vi "eyecat MAX v2-1_JS_160202.vi"() -> ()   [LabVIEW 2014]
doc: "This VI is an upgrade from the WIN 1_v4 that implements the ageing subrutine"
uses:
  Buttons/String output.ctl
  <vilib>/Utility/miscctls.llb/LVRowAndColumnTypeDef.ctl
  Buttons/Numeric control.ctl
  Buttons/String input.ctl
  Buttons/Numeric indicator.ctl
  Controls Win/Control 3.ctl
  <vilib>/Platform/TimedLoop/XDataNode/nitl_modes.ctl
  <vilib>/Platform/TimedLoop/XDataNode/timing_clust.ctl
  <vilib>/Platform/TimedLoop/XDataNode/wakeup.ctl
  <vilib>/Utility/file.llb/Write To Spreadsheet File (string).vi
  <vilib>/Utility/file.llb/Read From Spreadsheet File (string).vi
  <vilib>/Utility/file.llb/Read From Spreadsheet File (DBL).vi
  <vilib>/regexp/Match Regular Expression.xnode
  <vilib>/Platform/TimedLoop/XDataNode/XDataNode.xnode
  <vilib>/Platform/TimedLoop/XDataNode/XDNodeRunTimeDep.lvlib
panel:
  in  "Alarm":bool
  in  "Analyser":bool
  in  "MFC":bool
  in  "System":bool
  in  "Ageing":bool
  in  "Performance":bool
  in  "Home":bool
  out "NO":dbl[](array[numeric])
  out "CO":dbl[](array[numeric])
  out "MKS":bool
  out "7170":bool
  out "Pressure":dbl
  in  "Duration -1":i32
  in  "Demo Sync":i32
  in  "Demo On":bool
  in  "FlowGuide":bool
  in  "Mean(Off)/Interval(On) 2":bool
  in  "Flow Band %":dbl=1.04
  in  "Flow Sync":i32
  in  "Execute Leak Test Button":bool
  out "Emissions":dbl[](array[numeric])
  in  "Temperature Sync":i32
  in  "TempGuide":bool
  in  "Temp Band %":dbl=1.04
  in  "Mean(Off)/Interval(On)":bool
  in  "MKS 5Hz":bool
  out "output cluster":T2
  out "Lambda":dbl[](array[numeric])
  out "MKS HC":dbl
  in  "HC Index":i32
  in  "MFC Number":i32
  out "Open/Closed \nLoop":dbl[](array[numeric])
  out "Air Cyc 2":dbl[](array[numeric])
  in  "Cycle size":i32
  out "MFC Setpoint/Delivery":dynamicdata(graph)
  out "ExtAnDn":bool
  out "ExtAnUp":bool
  out "HC Cyc 2":dbl[](array[numeric])
  out "SO Valve 2":dbl[](array[numeric])
  out "SO Valve 1":dbl[](array[numeric])
  out "Air Bal":dbl[](array[numeric])
  out "HC Bal":dbl[](array[numeric])
  out "Air Cyc 1":dbl[](array[numeric])
  out "HC Cyc 1":dbl[](array[numeric])
  out "File name":string
  out "Log?":bool
  out "Advanced Logging":bool
  out "Connected":bool
  out "Furnace temp 2":dbl
  out "Full system?":bool
  out "Log interval (seconds)":T1
  in  "Flow rate Age":dbl
  in  "Inlet temp Age":dbl
  out "Stopped?":bool
  in  "Stop Cmd":T1
  out "Connected?":bool
  out "Error":dbl
  out "Iteration Duration":i64
  out "Finished Late? [i-1]":bool
  out "Furnace temp 1":dbl
  out "stop 2":bool
  in  "Enum 1":i16=1
  in  "Acknowledge":bool
  out "Test number":u16
  out "Flag1":bool=TRUE
  out "EditPos Subc":T3
  out "Flag 2":bool=TRUE
  in  "Tab Control":T4(tab)
  out "Warm Up":bool
  in  "Leak Test":bool
  in  "Stop Test":bool
  in  "Log Test Data":bool
  in  "Start Test":bool
  in  "Adv Settings":bool
  out "Doors Unlocked":bool
  in  "Temperature Limit (°C)":T1=1200.0 min=0.0 max=1200.0 step=1.0
  in  "File Name":T5="Test"
  in  "File Path":path=path "C:/DATA LOG"
  out "Fail":bool
  out "Pass":bool
  in  "Select Test Type":T6(radio)
  out "Standby":bool
  out "Doors Open":bool
  out "Extractor Fan On":bool
  out "Test In Progress":bool
  out "Cool Down":bool
  out "System Alarm":bool
  in  "Inlet Temperature (°C)":T1=400.0 min=350.0 max=1000.0 step=1.0
  in  "Inlet LAMBDA Rich":T1=0.9 min=0.85 max=0.96 step=0.001
  in  "Inlet LAMBDA Lean":T1=1.2 min=1.02 max=3.0 step=0.001
  in  "Test Stop temperature (°C)":T1=300.0 min=100.0 max=1000.0 step=1.0
  in  "Test Start Temperature (°C)":T1=125.0 min=0.0 max=500.0 step=1.0
  in  "Furnace Ramp Rate (°C/min)":T1=15.0 min=1.0 max=50.0 step=0.1
  in  "NO:CO Ratio":T1=1.1 min=1.0 max=5.0 step=0.1
  in  "Inlet O2 (%)":T1=0.5 min=0.0 max=14.0 step=0.01
  in  "Inlet LAMBDA":T1=1.0 min=0.6 max=3.0 step=0.001
  out "Space Velocity (h-1)":T7
  out "Vol Flow @ STP (l/min)":T7
  in  "Test Flow Rate(g/s)":T1 min=0.0 max=100.0 step=0.01
  out "Sample Volume (litres)":T7
  in  "Number of Samples":T1=1.0 min=1.0 max=6.0 step=1.0
  in  "Sample Diameter (mm)":T1
  out "CO Theory (%)":T7 format="%#_3g"
  out "CO Theory (%)":T7 format="%#_3g"
  out "HC Theory (%)":T7
  in  "Sample Length (mm)":T1 min=0.0 step=0.5
  in  "NO ppm SW":dbl=500.0 caption="NO (ppm)" min=0.0 max=500.0 step=1.0
  in  "NO ppm Loff":T1 caption="NO ppm"
  in  "Delete sCycle":bool
  in  "Load sCycle":bool
  in  "Save sCycle":bool
  in  "Clear subcycle":bool
  in  "Clear Cycle Pattern":bool
  in  "Save Cycle":bool
  in  "Load Cycle":bool
  in  "Delete Cycle":bool
  out "Test Compiled":bool
  in  "Compile Test Button":bool
  in  "Sub-Cycle List":i32(listbox)=1
  in  "Cycle List":i32(listbox)=2
  out "Total Test Duration (hrs)":T8
  in  "Ageing Gas":enum32{"Radio Selection 1", "Radio Selection 2"}(radio)
  in  "Sub-Cycle Pattern":string[][](table) caption="Subcycle pattern"
  in  "Total Number of Cycles":T1=1.0 min=1.0 max=10000.0 step=1.0
  in  "Cycle Pattern":string[][](table)
  in  "Sub-Cycle Name":T5
  in  "Cycle Name":T5
  out "Heat Exchanger Temperatures (°C)":dynamicdata(graph)
  out "Flow Rate (g/s)":dynamicdata(graph)
  out "Sample Temperatures (°C)":dynamicdata(graph)
  out "System Temperatures (°C)":dynamicdata(graph)
  in  "Graph 1 Box":string(combo)="CO"
  in  "Graph 4 Box":string(combo)="NO"
  in  "Graph 3 Box":string(combo)="Air Cycle 1"
  in  "Graph 2 Box":string(combo)="HC Cycle 1"
  out "MFC Graph 4":dynamicdata(graph)
  out "MFC Graph 3":dynamicdata(graph)
  out "MFC Graph 1":dynamicdata(graph)
  out "MFC Graph 2":dynamicdata(graph)
  out "HC Concentration (ppm)":dynamicdata(graph)
  out "Lambda":dynamicdata(graph)
  out "O2/CO Concentration":dynamicdata(graph)
  out "NO Concentration (ppm)":dynamicdata(graph)
  in  "Purge System":bool
  in  "Alarm ack":bool
  in  "Clear log":bool
  out "Table":string[][](table)
  out "Soft Alarm":bool
  out "Hard Alarm":bool
  # "0 CO \n1 HC Cyc 1\n2 Air Cyc 1\n3 NO\n4 Air Bal\n5 HC Bal\n6 Air Cyc 2\n7 HC Cyc 2"
  # "1% = 0.01"
  # "Test Type"
  # "Test Commands"
  # "System Indicators"
  # "Leak Test"
  # "Catalyst Specification"
  # "Lightoff Settings"
  # "Furnace Lightoff Settings"
  # "Sweep Settings"
  # "CO/HC Lightoff Settings"
  # "0.96 < lambda < 0.85"
  # "1.02< lambda < 1.6"
  # "350 < Tinlet < 1000"
  # "NO Lightoff Settings"
  # "Flow Specification"
  # "Cycle Compiled"
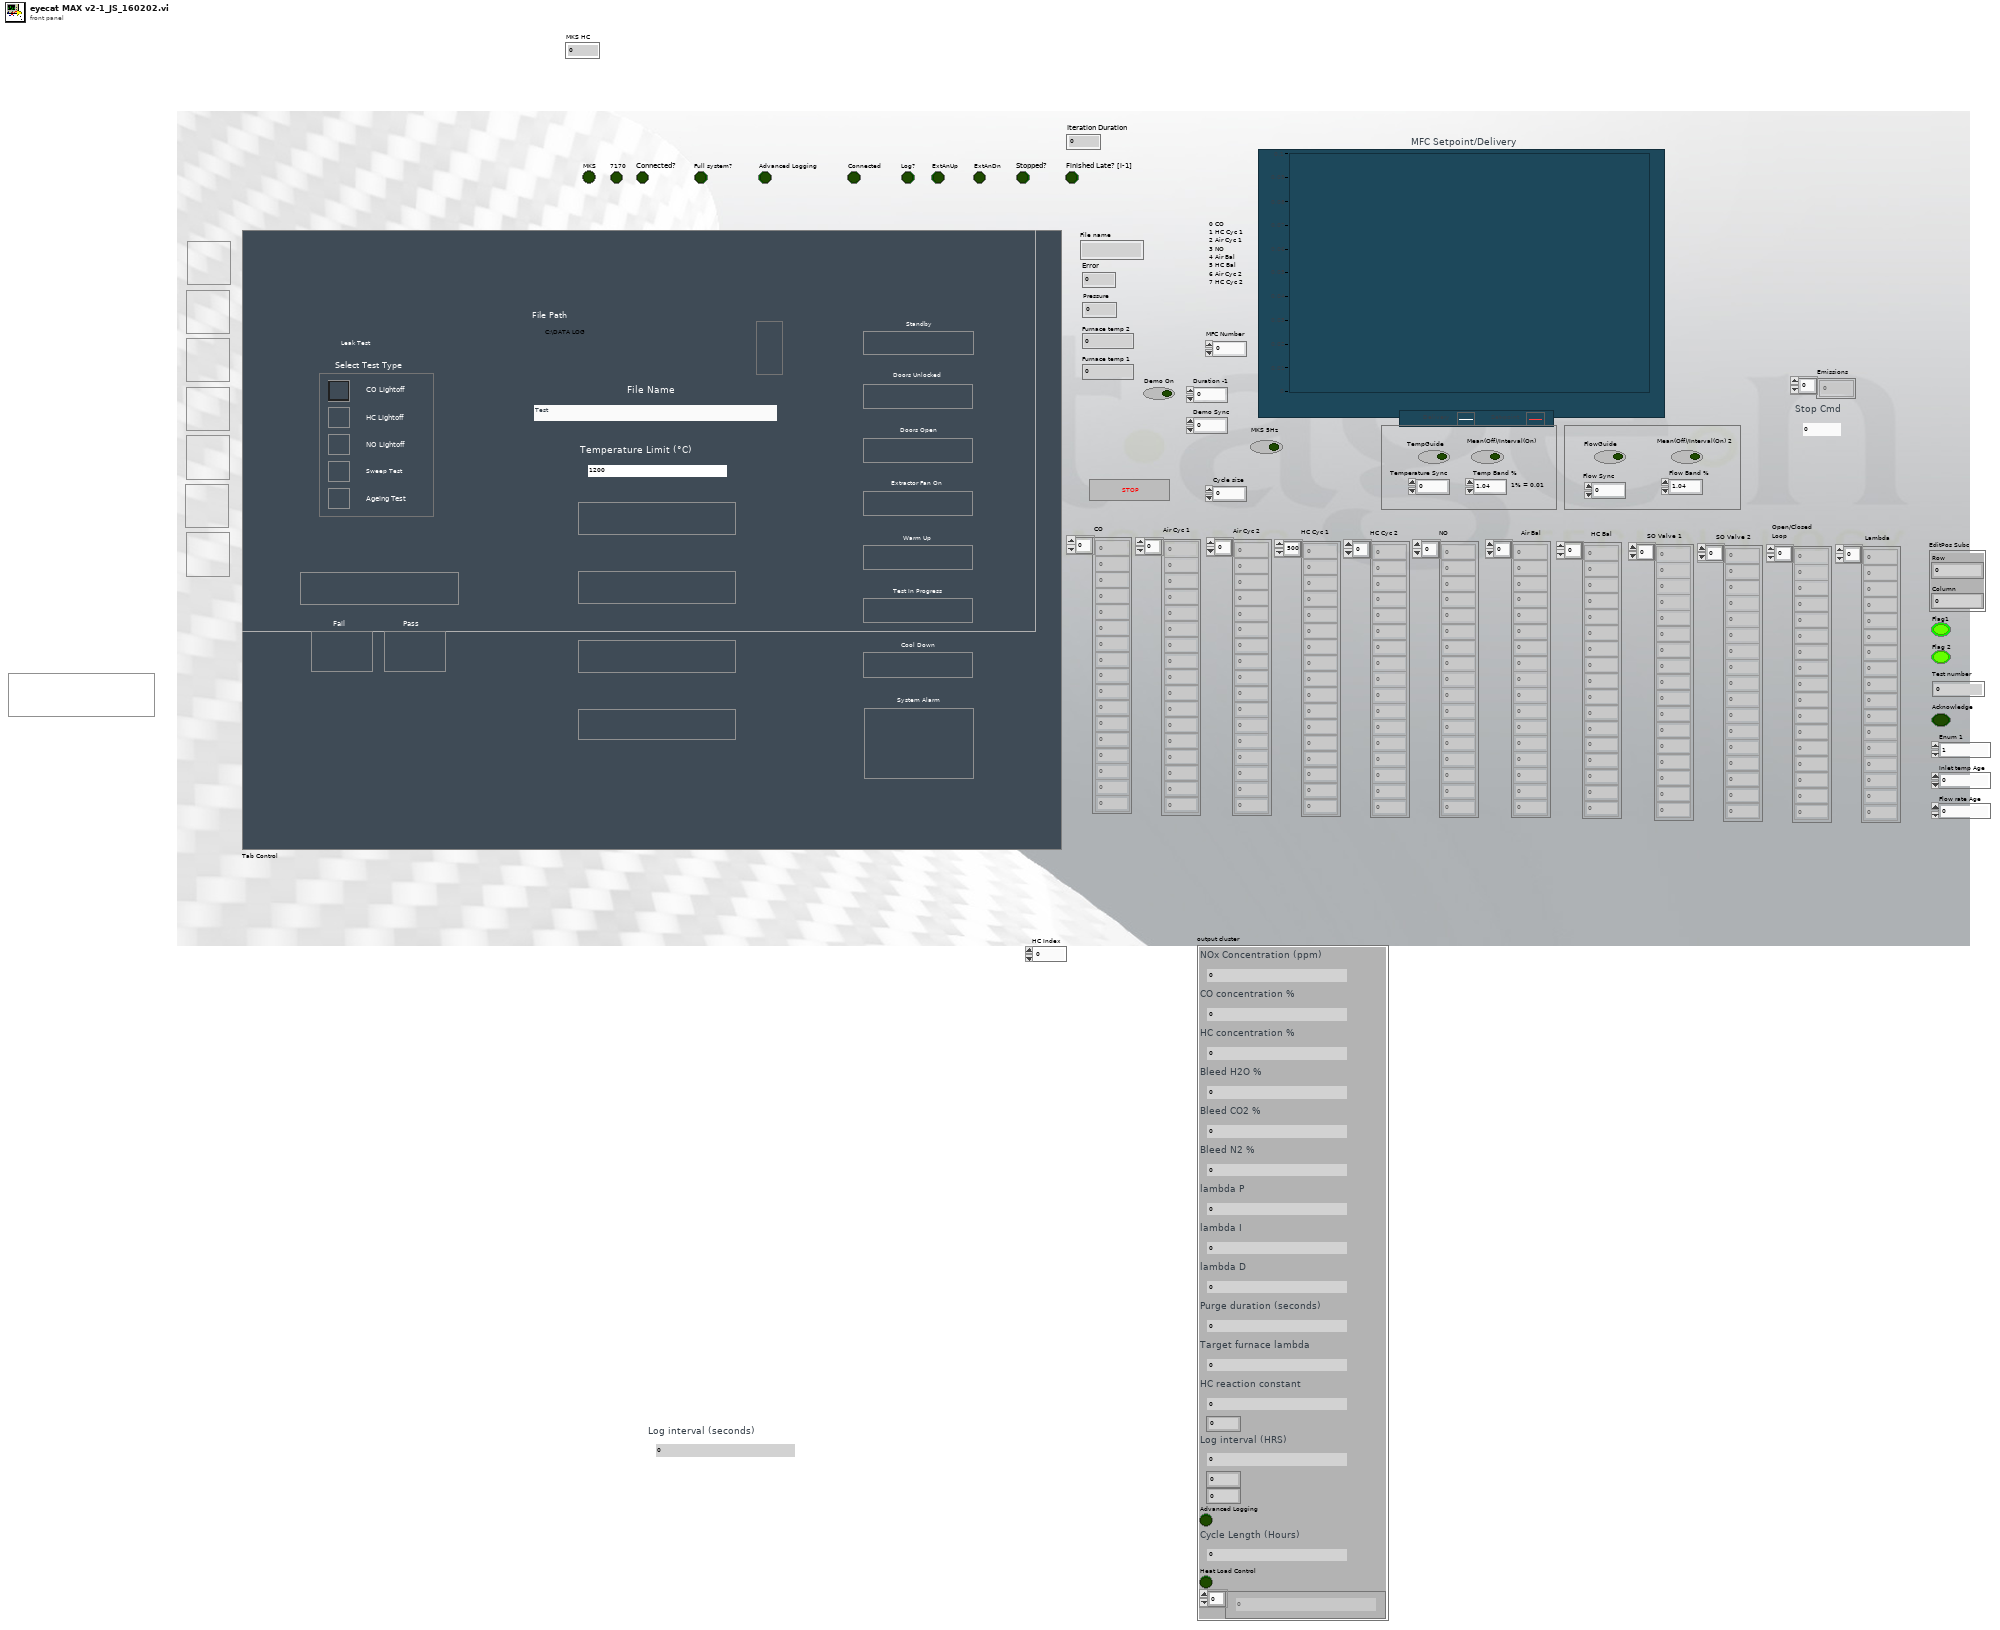
[diagram p1: front panel]
types:
  T1 = typedef "Numeric control.ctl" = dbl
  T2 = cluster{"NOx Concentration (ppm)":T1, "CO concentration %":T1, "HC concentration %":T1, "Bleed H2O %":T1, "Bleed CO2 %":T1, "Bleed N2 %":T1, "lambda P":T1, "lambda I":T1, "lambda D":T1, "Purge duration (seconds)":T1, "Target furnace lambda":T1, "HC reaction constant":T1, i16, "Log interval (HRS)":T1, i16, i16, "Advanced Logging":bool, "Cycle Length (Hours)":T1, "Heat Load Control":bool, T1[]}
  T3 = typedef "LVRowAndColumnTypeDef.ctl" = cluster{"Row":i32, "Column":i32}
  T4 = enum32{"MAIN", "PERFORMANCE TEST SETUP", "AGEING TEST SETUP", "SYSTEM DATA", "MFC", "ANALYSER DATA", "ALARM LOG"}
  T5 = typedef "String input.ctl" = string
  T6 = enum32{"CO Lightoff", "HC Lightoff", "NO Lightoff", "Sweep Test", "Ageing Test"}
  T7 = typedef "Numeric indicator.ctl" = dbl
  T8 = typedef "String output.ctl" = string
  T9 = typedef "XDNodeRunTimeDep.lvlib/nitl_modes.ctl" = enum32{"No Change", "Process missed periods, maintain original phase", "Discard missed periods, maintain original phase", "Process missed periods, ignore original phase", "Discard missed periods, ignore original phase"}
  T10 = typedef "Control 3.ctl" = enum16{"main", "start test", "save subc", "load subc", "delete subc", "clear table 1", "update list 1", "save cycle", "load cycle", "delete cycle", "clear table 2", "update list 2", "calc HC CO", "Total time calc", "update Cycle pattern ", "load cycle name", "convert to num", "load test array", "check scycle name", "check cycle name", "Multigas connect", "Multigas disconnect", "Leak Test"}
  T11 = enum8{"Enabled", "Disabled", "Disabled and Grayed Out"}
  T12 = typedef "XDNodeRunTimeDep.lvlib/timing_clust.ctl" = cluster{"Expected End [f-1]":u64, "Actual End [f-1]":u64, "Finished Late? [f-1]":bool, "Expected End [i-1]":u64, "Actual End [i-1]":u64, "Finished Late? [i-1]":bool, "Expected Start [i]":u64, "Actual Start [i]":u64, "Expected Start [f]":u64, "Actual Start [f]":u64, "Source Name":string, "Structure Name":string, "Period":i64, "Deadline":i64, "Offset":i64, "Start":i64, "Priority":i32, "Timeout":i32, "Mode":T9, "Wakeup Reason":T13, "Error":errorcluster, "Source Type":string, "Secondary Source Type":string, "Global End Time":u64, "Global Start Time":u64, "Frame Duration":u64, "Iteration Duration":u64, "Assigned CPU":i32, "I/O Scan Engine Mode":u32}
  T13 = typedef "XDNodeRunTimeDep.lvlib/wakeup.ctl" = enum32{"Normal", "Aborted", "Asynchronous wakeup", "Timing source error", "Timed loop error", "Timeout"}
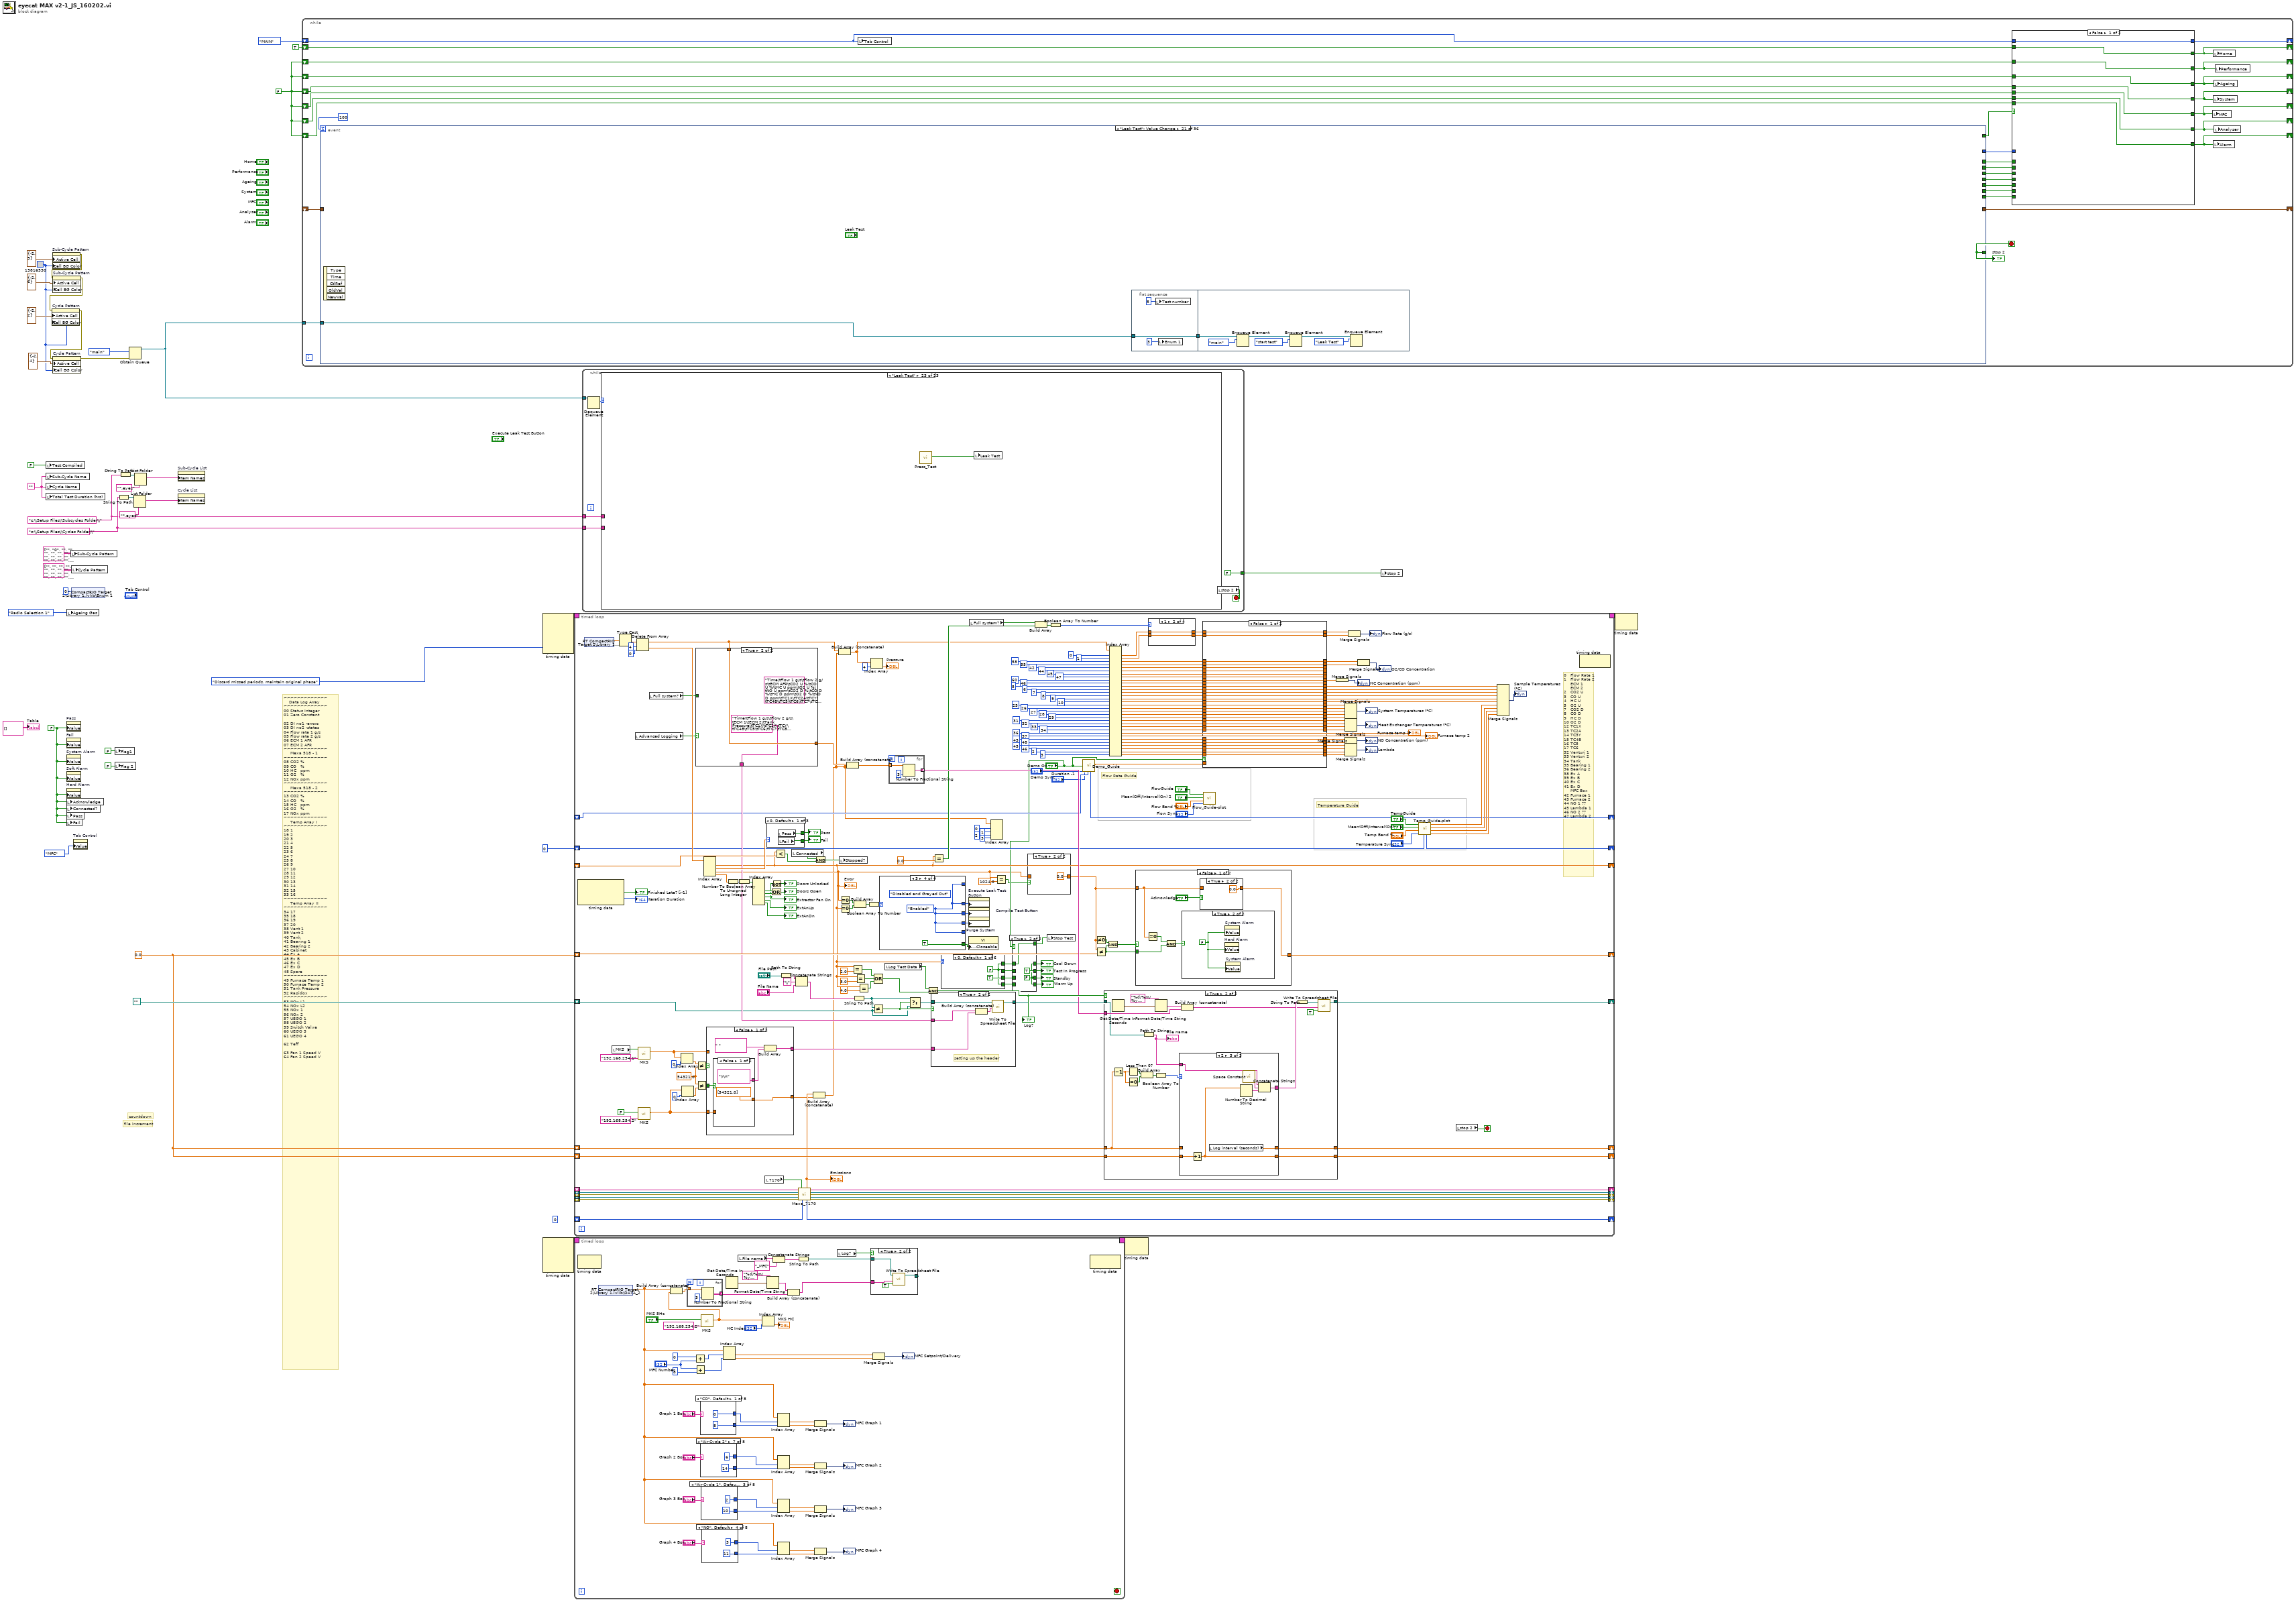
[diagram p0: block diagram]
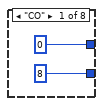
[diagram p2: hidden frame]
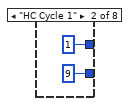
[diagram p3: hidden frame]
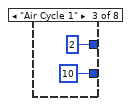
[diagram p4: hidden frame]
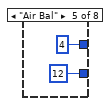
[diagram p5: hidden frame]
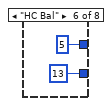
[diagram p6: hidden frame]
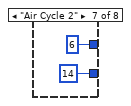
[diagram p7: hidden frame]
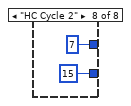
[diagram p8: hidden frame]
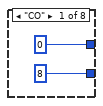
[diagram p9: hidden frame]
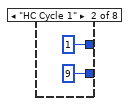
[diagram p10: hidden frame]
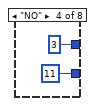
[diagram p11: hidden frame]
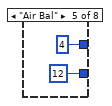
[diagram p12: hidden frame]
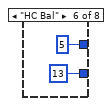
[diagram p13: hidden frame]
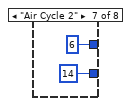
[diagram p14: hidden frame]
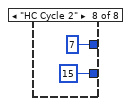
[diagram p15: hidden frame]
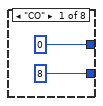
[diagram p16: hidden frame]
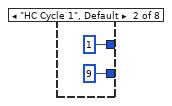
[diagram p17: hidden frame]
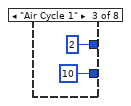
[diagram p18: hidden frame]
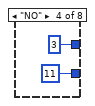
[diagram p19: hidden frame]
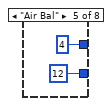
[diagram p20: hidden frame]
diagram:
  w1 = FALSE
  (unwired) 0 ("index")
  w9 = FALSE
  w8 = 0.0 ("y")
  w24 = ""
  w27 = "c:\\Setup Files\\Cycles Folder\\"
  w33 = u32 13816530
  w25 = "c:\\Setup Files\\Subcycles Folder\\"
  # "~~~~~~~~~~~~~\n    Data Log Array\n~~~~~~~~~~~~~\n00 Status Integer\n01 Zero Constant\n\n02 DI no1 -errors\n03 DI no2 -states\n04 Flow rate 1 g/s\n05 Flow rate 2 g/s\n06 ECM 1 AFR\n07 ECM 2 AFR\n~~~~~~~~~~~~~\n     Mexa 518 - 1\n~~~~~~~~~~~~~\n08 CO2 %\n09 CO   %\n10 HC   ppm\n11 O2   %\n12 NOx ppm\n~~~~~~~~~~~~~\n     Mexa 518 - 2\n~~~~~~~~~~~~~\n13 CO2 %\n14 CO   %\n15 HC   ppm\n16 O2   %\n17 NOx ppm\n~~~~~~~~~~~~~\n     Temp Array I\n~~~~~~~~~~~~~\n18 1\n19 2 \n20 3\n21 4\n22 5\n23 6\n24 7\n25 8\n26 9\n27 10\n28 11\n29 12\n30 13\n31 14\n32 15\n33 16\n~~~~~~~~~~~~~\n     Temp Array II\n~~~~~~~~~~~~~\n34 17\n35 18\n36 19\n37 20\n38 Vent 1\n39 Vent 2\n40 Tank\n41 Bearing 1\n42 Bearing 2\n43 Cabinet\n44 Ex A\n45 Ex B\n46 Ex C\n47 Ex D\n48 Spare\n~~~~~~~~~~~~~\n49 Furnace Temp 1\n50 Furnace Temp 2\n51 Tank Pressure\n52 Rapidox\n~~~~~~~~~~~~~\n53 NOx L1\n54 NOx L2\n55 NOx 1\n56 NOx 2\n57 UEGO 1\n58 UEGO 2\n59 Switch Valve\n60 UEGO 3\n61 UEGO 4\n\n62 Teff\n\n63 Fan 1 Speed V\n64 Fan 2 Speed V"
  # "file increment"
  # "countdown"
  n1 = local write "Test Compiled"(FALSE ("Cycle Compiled")) -> ()
  n2 = local write "Sub-Cycle Name"(w24) -> ()
  n3 = local write "Cycle Name"(w24) -> ()
  n4 = local write "Total Test Duration (hrs)"(w24) -> ()
  n5 = property on="Sub-Cycle Pattern" class="Tbl (strict)"("Active Cell"=T3 {"Row"=-2, "Column"=5} ("Active Cell:Active Cell"), "Cell BG Color"=w33) -> (error out=w38:errorcluster)  [unwired: 2 in, 1 out]
  n6 = property on="Sub-Cycle Pattern" class="Tbl (strict)"(error in=w38, "Active Cell"=T3 {"Row"=-2, "Column"=6} ("Active Cell:Active Cell"), "Cell BG Color"=w33) -> (error out=w37:errorcluster)  [unwired: 1 in, 1 out]
  n7 = property on="Cycle Pattern" class="Tbl (strict)"(error in=w37, "Active Cell"=T3 {"Row"=-2, "Column"=2} ("Active Cell:Active Cell"), "Cell BG Color"=w33) -> (error out=w35:errorcluster)  [unwired: 1 in, 1 out]
  n8 = property on="Cycle Pattern" class="Tbl (strict)"(error in=w35, "Active Cell"=T3 {"Row"=-2, "Column"=4} ("Active Cell:Active Cell"), "Cell BG Color"=w33) -> (error out=w32:errorcluster)  [unwired: 1 in, 1 out]
  n9 = property on="Pass" class="Bool (strict)"("Value"=w9) -> ()  [unwired: 2 in, 2 out]
  n10 = property on="Fail" class="Bool (strict)"("Value"=w9) -> ()  [unwired: 2 in, 2 out]
  n11 = property on="System Alarm" class="Bool (strict)"("Value"=w9) -> ()  [unwired: 2 in, 2 out]
  n12 = property on="Soft Alarm" class="Bool (strict)"("Value"=w9) -> ()  [unwired: 2 in, 2 out]
  n13 = property on="Hard Alarm" class="Bool (strict)"("Value"=w9) -> ()  [unwired: 2 in, 2 out]
  n14 = local write "Acknowledge"(w9) -> ()
  n15 = local write "Connected?"(w9) -> ()
  n16 = local write "Pass"(w9) -> ()
  n17 = local write "Fail"(w9) -> ()
  n18 = local write "Ageing Gas"(enum32{"Radio Selection 1", "Radio Selection 2"}."Radio Selection 1" ("Ageing Gas")) -> ()
  n19 = local write "Sub-Cycle Pattern"(string[][] [["", "0", "", "", "", "", "", "", "", "", "", "", ""], ["", "", "", "", "", "", "", "", "", "", "", "", ""], ["", "", "", "", "", "", "", "", "", "", "", "", ""], ["", "", "", "", "", "", "", "", "", "", "", "", ""], ["", "", "", "", "", "", "", "", "", "", "", "", ""], ["", "", "", "", "", "", "", "", "", "", "", "", ""], ["", "", "", "", "", "", "", "", "", "", "", "", ""], ["", "", "", "", "", "", "", "", "", "", "", "", ""], ["", "", "", "", "", "", "", "", "", "", "", "", ""], ["", "", "", "", "", "", "", "", "", "", "", "", ""], ["", "", "", "", "", "", "", "", "", "", "", "", ""], ["", "", "", "", "", "", "", "", "", "", "", "", ""], ["", "", "", "", "", "", "", "", "", "", "", "", ""], ["", "", "", "", "", "", "", "", "", "", "", "", ""], ["", "", "", "", "", "", "", "", "", "", "", "", ""], ["", "", "", "", "", "", "", "", "", "", "", "", ""], ["", "", "", "", "", "", "", "", "", "", "", "", ""], ["", "", "", "", "", "", "", "", "", "", "", "", ""], ["", "", "", "", "", "", "", "", "", "", "", "", ""], ["", "", "", "", "", "", "", "", "", "", "", "", ""], ["", "", "", "", "", "", "", "", "", "", "", "", ""], ["", "", "", "", "", "", "", "", "", "", "", "", ""], ["", "", "", "", "", "", "", "", "", "", "", "", ""], ["", "", "", "", "", "", "", "", "", "", "", "", ""], ["", "", "", "", "", "", "", "", "", "", "", "", ""], ["", "", "", "", "", "", "", "", "", "", "", "", ""], ["", "", "", "", "", "", "", "", "", "", "", "", ""], ["", "", "", "", "", "", "", "", "", "", "", "", ""], ["", "", "", "", "", "", "", "", "", "", "", "", ""], ["", "", "", "", "", "", "", "", "", "", "", "", ""], ["", "", "", "", "", "", "", "", "", "", "", "", ""]]) -> ()
  n20 = local write "Cycle Pattern"(string[][] [["", "", "", "", ""], ["", "", "", "", ""], ["", "", "", "", ""], ["", "", "", "", ""], ["", "", "", "", ""], ["", "", "", "", ""], ["", "", "", "", ""], ["", "", "", "", ""], ["", "", "", "", ""], ["", "", "", "", ""], ["", "", "", "", ""], ["", "", "", "", ""], ["", "", "", "", ""], ["", "", "", "", ""], ["", "", "", "", ""], ["", "", "", "", ""], ["", "", "", "", ""], ["", "", "", "", ""], ["", "", "", "", ""], ["", "", "", "", ""], ["", "", "", "", ""], ["", "", "", "", ""], ["", "", "", "", ""], ["", "", "", "", ""], ["", "", "", "", ""], ["", "", "", "", ""], ["", "", "", "", ""], ["", "", "", "", ""], ["", "", "", "", ""], ["", "", "", "", ""], ["", "", "", "", ""]]) -> ()
  n21 = shared-variable "RT CompactRIO Target 2\\Library 1.lvlib\\Enum 1"(u16 0 ("Enum 1")) -> ()  [unwired: 1 in, 1 out]
  n22 = property on="Tab Control" class="TabCtl (strict)"("Value"=T4."MFC" ("Tab Control")) -> ()  [unwired: 2 in, 2 out]
  n23 = local write "Flag1"(FALSE) -> ()
  n24 = local write "Flag 2"(FALSE) -> ()
  n25 = String To Path(string=w27) -> (path=w28:path)
  n26 = String To Path(string=w25) -> (path=w30:path)
  n27 = Obtain Queue(element data type=Control_3."main" ("Enum"), error in (no error)=w32) -> (queue out=w41:refnum<queue>)  [unwired: 3 in, 2 out]
  n28 = List Folder(path=w28, pattern="*.eyec") -> (filenames=w29:string[])  [unwired: 2 in, 3 out]
  n29 = List Folder(path=w30, pattern="*.eyes") -> (filenames=w31:string[])  [unwired: 2 in, 3 out]
  n30 = property on="Sub-Cycle List" class="LstBox (strict)"("Item Names"=w31) -> ()  [unwired: 2 in, 2 out]
  n31 = property on="Cycle List" class="LstBox (strict)"("Item Names"=w29) -> ()  [unwired: 2 in, 2 out]
  n32 = while {
    tunnel: w41 -> [w72]
    shift-right: [w70] -> _
    shift-left: _ -> [w69]
    shift-right: [w67] -> _
    shift-left: T4."MAIN" ("Tab Control") -> [w66]
    shift-right: [w55] -> _
    shift-left: w1 -> [w48]
    shift-right: [w56] -> _
    shift-left: TRUE -> [w49]
    shift-right: [w54] -> _
    shift-left: w1 -> [w43]
    shift-right: [w53] -> _
    shift-left: w1 -> [w44]
    shift-right: [w52] -> _
    shift-left: w1 -> [w45]
    shift-right: [w51] -> _
    shift-left: w1 -> [w46]
    shift-right: [w50] -> _
    shift-left: w1 -> [w47]
    stop <- w68 stop-if-true
    n33 = event shown="[20] \"Leak Test\": Value Change" {
      selector: _ -> [_ _ _ _ _ _ _ _ _ _ _ _ _ _ _ _ _ _ _ _ _ _ _ _ _ _ _ _ _ _ _ _ _ _ _ _]
      dyn-events: _ -> [_ _ _ _ _ _ _ _ _ _ _ _ _ _ _ _ _ _ _ _ _ _ _ _ _ _ _ _ _ _ _ _ _ _ _ _]
      timeout: 100 -> [_ _ _ _ _ _ _ _ _ _ _ _ _ _ _ _ _ _ _ _ _ _ _ _ _ _ _ _ _ _ _ _ _ _ _ _]
      tunnel: w72 -> [w91 w93 _ w102 w110 w117 w124 w135 w139 w150 w155 w158 w163 w185 w193 w194 _ _ _ _ w238 w249 _ w341 w365 _ w379 _ _ _ _ _ _ _ _ _]
      tunnel: [w89 w92 _ w103 w109 w116 w123 w134 w137 w145 w152 w157 w161 w182 _ _ _ _ _ _ _ _ _ _ _ _ _ _ _ _ _ _ _ _ _ _] -> w70
      tunnel: w69 -> [w89 w92 _ w103 w109 w116 w122 w134 w137 w145 w152 w157 w161 w182 _ _ _ _ _ _ _ _ _ _ _ _ _ _ _ _ _ _ _ _ _ _]
      tunnel: [_ _ w95 _ _ _ _ _ _ _ _ _ _ _ _ _ _ _ _ _ _ _ _ _ _ _ _ _ _ _ _ _ _ _ _ _] -> w68
      tunnel: [_ _ _ _ _ _ _ _ _ _ _ _ _ _ _ _ _ _ _ _ _ _ _ _ _ _ _ _ _ TRUE TRUE TRUE TRUE TRUE TRUE TRUE] -> w65
      tunnel: [_ _ _ _ _ _ _ _ _ _ _ _ _ _ _ _ _ _ _ _ _ _ _ _ _ _ _ _ _ T4."MAIN" ("Tab Control") T4."PERFORMANCE TEST SETUP" ("Tab Control") T4."AGEING TEST SETUP" ("Tab Control") T4."SYSTEM DATA" ("Tab Control") T4."MFC" ("Tab Control") T4."ANALYSER DATA" ("Tab Control") T4."ALARM LOG" ("Tab Control")] -> w64
      tunnel: [_ _ _ _ _ _ _ _ _ _ _ _ _ _ _ _ _ _ _ _ _ _ _ _ _ _ _ _ _ TRUE w390 w394 w398 w402 w407 w410] -> w63
      tunnel: [_ _ _ _ _ _ _ _ _ _ _ _ _ _ _ _ _ _ _ _ _ _ _ _ _ _ _ _ _ w387 TRUE w394 w398 w402 w407 w410] -> w62
      tunnel: [_ _ _ _ _ _ _ _ _ _ _ _ _ _ _ _ _ _ _ _ _ _ _ _ _ _ _ _ _ w387 w390 TRUE w398 w402 w407 w410] -> w61
      tunnel: [_ _ _ _ _ _ _ _ _ _ _ _ _ _ _ _ _ _ _ _ _ _ _ _ _ _ _ _ _ w387 w390 w394 TRUE w402 w407 w410] -> w60
      tunnel: [_ _ _ _ _ _ _ _ _ _ _ _ _ _ _ _ _ _ _ _ _ _ _ _ _ _ _ _ _ w387 w390 w394 w398 TRUE w407 w410] -> w59
      tunnel: [_ _ _ _ _ _ _ _ _ _ _ _ _ _ _ _ _ _ _ _ _ _ _ _ _ _ _ _ _ w387 w390 w394 w398 w402 TRUE w410] -> w58
      tunnel: [_ _ _ _ _ _ _ _ _ _ _ _ _ _ _ _ _ _ _ _ _ _ _ _ _ _ _ _ _ w387 w390 w394 w398 w402 w407 TRUE] -> w57
      event Timeout {
        n34 = event-data() -> ()  [unwired: 1 in, 2 out]
        n35 = Enqueue Element(queue=w91, element=Control_3."main" ("Enum")) -> ()  [unwired: 2 in, 3 out]
      }
      event "Clear subcycle": Value Change {
        n36 = event-data() -> ()  [unwired: 1 in, 5 out]
        n37 = Enqueue Element(queue=w93, element=Control_3."clear table 1" ("Enum")) -> ()  [unwired: 2 in, 3 out]
      }
      event Panel Close? {
        n38 = event-data() -> ()  [unwired: 1 in, 3 out]
        n39 = Two Button Dialog(message="This command will close Eyecat!\nDo you wish to continue?", 1:"No" ("F button name (\"Cancel\")"), 2:"Yes" ("T button name (\"OK\")")) -> (T button?=w95:bool)
        n40 = Not(x=w95) -> (.not. x?=w96:bool)
        n41 = event-data("Discard?"=w96) -> ()  [unwired: 1 in, 1 out]
      }
      event "Save sCycle": Value Change {
        n42 = event-data() -> ()  [unwired: 1 in, 5 out]
        n43 = local read "Sub-Cycle Pattern"() -> (w100:string[][])
        n44 = call "Time column check.vi"("Array"=w100) -> ("Mistake?"=w101:bool)  [unwired: 10 in]
        n45 = case shown="False" w101 {
          tunnel: w102 -> [w104 _]
          frame False {
            n46 = Enqueue Element(queue=w104, element=Control_3."save subc") -> (queue out=w106:refnum<queue>)  [unwired: 2 in, 2 out]
            n47 = Enqueue Element(queue=w106, element=Control_3."update list 1") -> ()  [unwired: 2 in, 3 out]
          }
          frame True {
            n48 = One Button Dialog(message="The time sequence is incorrect!\nReview and save again!") -> ()  [unwired: 1 in, 1 out]
          }
        }
      }
      event "Load sCycle": Value Change {
        n49 = event-data() -> ()  [unwired: 1 in, 5 out]
        n50 = Enqueue Element(queue=w110, element=Control_3."load subc") -> ()  [unwired: 2 in, 3 out]
      }
      event "Delete sCycle": Value Change {
        n51 = event-data() -> ()  [unwired: 1 in, 5 out]
        n52 = Enqueue Element(queue=w117, element=Control_3."delete subc") -> (queue out=w119:refnum<queue>)  [unwired: 2 in, 2 out]
        n53 = Enqueue Element(queue=w119, element=Control_3."update list 1") -> (queue out=w115:refnum<queue>)  [unwired: 2 in, 2 out]
        n54 = Enqueue Element(queue=w115, element=Control_3."update Cycle pattern ") -> (queue out=w112:refnum<queue>)  [unwired: 2 in, 2 out]
        n55 = Enqueue Element(queue=w112, element=Control_3."Total time calc") -> ()  [unwired: 2 in, 3 out]
      }
      event "Sub-Cycle Pattern": Mouse Down; "Sub-Cycle Pattern": Value Change {
        n56 = event-data() -> ()  [unwired: 1 in, 3 out]
        n57 = property on="Sub-Cycle Pattern" class="Tbl (strict)"() -> ("EditPos"=w123:T3)  [unwired: 2 in, 2 out]
        n58 = Unbundle By Name(w123) -> ("Row"=w125:i32)  [unwired: 1 out]
        n59 = Less?(x=w125, y=30) -> (x < y?=w127:bool)
        n60 = case shown="True" w127 {
          tunnel: w124 -> [_ w132]
          frame False {
            n61 = One Button Dialog(message="This table is limited to 30 entries!") -> ()  [unwired: 1 in, 1 out]
          }
          frame True {
            n62 = Enqueue Element(queue=w132, element=Control_3."convert to num") -> (queue out=w131:refnum<queue>)  [unwired: 2 in, 2 out]
            n63 = Enqueue Element(queue=w131, element=Control_3."calc HC CO") -> ()  [unwired: 2 in, 3 out]
          }
        }
        "EditPos Subc" <- w122
        "Flag1" <- TRUE
      }
      event "Clear Cycle Pattern": Value Change {
        n64 = event-data() -> ()  [unwired: 1 in, 5 out]
        n65 = Enqueue Element(queue=w135, element=Control_3."clear table 2" ("Enum")) -> ()  [unwired: 2 in, 3 out]
        n66 = local write "Test Compiled"(FALSE ("Test Compiled")) -> ()
      }
      event "Save Cycle": Value Change {
        n67 = event-data() -> ()  [unwired: 1 in, 5 out]
        n68 = Enqueue Element(queue=w139, element=Control_3."update Cycle pattern ") -> (queue out=w138:refnum<queue>)  [unwired: 2 in, 2 out]
        n69 = Enqueue Element(queue=w138, element=Control_3."save cycle") -> (queue out=w142:refnum<queue>)  [unwired: 2 in, 2 out]
        n70 = Enqueue Element(queue=w142, element=Control_3."update list 2") -> ()  [unwired: 2 in, 3 out]
      }
      event "Load Cycle": Value Change {
        n71 = event-data() -> ()  [unwired: 1 in, 5 out]
        n72 = Enqueue Element(queue=w150, element=Control_3."load cycle") -> (queue out=w148:refnum<queue>)  [unwired: 2 in, 2 out]
        n73 = Enqueue Element(queue=w148, element=Control_3."update Cycle pattern ") -> (queue out=w147:refnum<queue>)  [unwired: 2 in, 2 out]
        n74 = local write "Test Compiled"(FALSE ("Test Compiled")) -> ()
        n75 = Enqueue Element(queue=w147, element=Control_3."Total time calc") -> ()  [unwired: 2 in, 3 out]
      }
      event "Delete Cycle": Value Change {
        n76 = event-data() -> ()  [unwired: 1 in, 5 out]
        n77 = Enqueue Element(queue=w155, element=Control_3."delete cycle") -> (queue out=w154:refnum<queue>)  [unwired: 2 in, 2 out]
        n78 = Enqueue Element(queue=w154, element=Control_3."update list 2") -> ()  [unwired: 2 in, 3 out]
      }
      event Value Change {
        n79 = event-data() -> ()  [unwired: 1 in, 5 out]
        n80 = Enqueue Element(queue=w158, element=Control_3."Total time calc") -> ()  [unwired: 2 in, 3 out]
      }
      event "Cycle Pattern": Mouse Up; "Cycle Pattern": Value Change {
        n81 = event-data() -> ()  [unwired: 1 in, 3 out]
        n82 = property on="Cycle Pattern" class="Tbl (strict)"() -> ("EditPos"=w165:T3)  [unwired: 2 in, 2 out]
        n83 = Unbundle By Name(w165) -> ("Row"=w162:i32, "Column"=w167:i32)
        n84 = Less?(x=w162, y=30) -> (x < y?=w166:bool)
        n85 = case shown="True" w166 {
          tunnel: w167 -> [_ w169]
          tunnel: w163 -> [_ w172]
          frame False {
            n86 = One Button Dialog(message="This table is limited to 30 entries!") -> ()  [unwired: 1 in, 1 out]
          }
          frame True {
            n87 = Equal?(x=w169, y=1) -> (x = y?=w173:bool)
            n88 = case shown="True" w173 {
              tunnel: w172 -> [w176 w179]
              tunnel: [w175 w178] -> w171
              frame False {
                n89 = Enqueue Element(queue=w176, element=Control_3."update Cycle pattern ") -> (queue out=w175:refnum<queue>)  [unwired: 2 in, 2 out]
              }
              frame True {
                n90 = Enqueue Element(queue=w179, element=Control_3."load cycle name") -> (queue out=w178:refnum<queue>)  [unwired: 2 in, 2 out]
              }
            }
            n91 = Enqueue Element(queue=w171, element=Control_3."Total time calc") -> ()  [unwired: 2 in, 3 out]
          }
        }
        "Flag 2" <- TRUE
      }
      event "Compile Test Button": Value Change {
        n92 = event-data() -> ()  [unwired: 1 in, 5 out]
        n93 = local read "Flag 2"() -> (w181:bool)
        n94 = case shown="True" w181 {
          tunnel: w185 -> [w186 w190]
          tunnel: [w186 w187] -> w183
          frame False {
          }
          frame True {
            n95 = Enqueue Element(queue=w190, element=Control_3."save cycle") -> (queue out=w188:refnum<queue>)  [unwired: 2 in, 2 out]
            n96 = Enqueue Element(queue=w188, element=Control_3."update list 2") -> (queue out=w187:refnum<queue>)  [unwired: 2 in, 2 out]
          }
        }
        n97 = Enqueue Element(queue=w183, element=Control_3."load test array") -> ()  [unwired: 2 in, 3 out]
      }
      event Value Change {
        n98 = event-data() -> ()  [unwired: 1 in, 5 out]
        n99 = Enqueue Element(queue=w193, element=Control_3."check scycle name") -> ()  [unwired: 2 in, 3 out]
      }
      event Value Change {
        n100 = event-data() -> ()  [unwired: 1 in, 5 out]
        n101 = Enqueue Element(queue=w194, element=Control_3."check cycle name") -> ()  [unwired: 2 in, 3 out]
      }
      event Value Change {
        n102 = event-data() -> ()  [unwired: 1 in, 5 out]
        n103 = Square(x="Sample Diameter (mm)") -> (x^2=w203:T1)
        n104 = Compound Arithmetic op=MULTIPLY(w203, "Sample Length (mm)", "Number of Samples", 3.141592653589793) -> (w202:T1)
        n105 = Divide(x=w202, y=4000000.0) -> (x/y=→"Sample Volume (litres)":T1)
      }
      event Value Change {
        # "O2Eq"
        n106 = event-data() -> ()  [unwired: 1 in, 5 out]
        n107 = local write "Inlet LAMBDA"("Inlet LAMBDA") -> ()
        n108 = local write "Inlet O2 (%)"("Inlet O2 (%)") -> ()
        n109 = Decrement(x="Inlet LAMBDA") -> (x-1=w218:T1)
        n110 = Multiply(x=4.76, y="Inlet LAMBDA") -> (x*y=w214:T1)
        n111 = Multiply(x=w218, y=100.0) -> (x*y=w216:T1)
        n112 = Add(x=0.33, y=w214) -> (x+y=w212:T1)
        n113 = Divide(x=w216, y=w212) -> (x/y=w211:T1)
        n114 = Subtract(x="Inlet O2 (%)", y=w211) -> (x-y=w209:T1)
        n115 = Multiply(x=w209, y=2.0) -> (x*y=→"CO Theory (%)":T1)
        n116 = Divide(x=w209, y=4.5) -> (x/y=→"HC Theory (%)":T1)
      }
      event Value Change {
        n117 = event-data() -> ()  [unwired: 1 in, 5 out]
        n118 = local write "NO ppm Loff"("NO ppm Loff") -> ()
        n119 = local write "NO:CO Ratio"("NO:CO Ratio") -> ()
        n120 = Divide(x="NO ppm Loff", y=T1 10000.0) -> (x/y=w221:T1)
        n121 = Multiply(x="NO:CO Ratio", y=w221) -> (x*y=→"CO Theory (%)":T1)
      }
      event Value Change {
        n122 = event-data() -> ()  [unwired: 1 in, 5 out]
        n123 = local read "Sample Volume (litres)"() -> (w226:T7)
        n124 = Equal?(x=w226, y=0.0) -> (x = y?=w225:bool)
        n125 = case shown="False" w225 {
          tunnel: w226 -> [w231 _]
          tunnel: "Test Flow Rate(g/s)" -> [w228 _]
          frame False {
            w233 = 60.0 ("y")
            n126 = Multiply(x=w228, y=w233) -> (x*y=w235:T1)
            n127 = Divide(x=w235, y=1.2) -> (x/y=w230:T1)
            "Vol Flow @ STP (l/min)" <- w230
            n128 = Multiply(x=w230, y=w233) -> (x*y=w232:T1)
            n129 = Divide(x=w232, y=w231) -> (x/y=→"Space Velocity (h-1)":T1)
          }
          frame True {
            n130 = One Button Dialog(message="Review sample specification first!") -> ()  [unwired: 1 in, 1 out]
          }
        }
      }
      event "Leak Test": Value Change {
        n131 = event-data() -> ()  [unwired: 1 in, 5 out]
        n132 = flat-sequence {
          tunnel: w238 -> [w241]
          tunnel: [w241] -> w237
          tunnel: w237 -> [w246]
          frame #0 {
            n133 = local write "Test number"(u16 5) -> ()
            n134 = local write "Enum 1"(u16 3 ("Test number")) -> ()
          }
          frame #1 {
            n135 = Enqueue Element(queue=w246, element=Control_3."main" ("Enum")) -> (queue out=w244:refnum<queue>)  [unwired: 2 in, 2 out]
            n136 = Enqueue Element(queue=w244, element=Control_3."start test" ("Enum")) -> (queue out=w243:refnum<queue>)  [unwired: 2 in, 2 out]
            n137 = Enqueue Element(queue=w243, element=Control_3."Leak Test" ("Enum")) -> ()  [unwired: 2 in, 3 out]
          }
        }
      }
      event "Start Test": Value Change {
        n138 = event-data() -> ()  [unwired: 1 in, 6 out]
        n139 = case shown="True" "Start Test" {
          tunnel: w249 -> [_ w258]
          frame False {
          }
          frame True {
            n140 = local read "Log Test Data"() -> (w250:bool)
            n141 = Boolean To (0,1)(Boolean=w250) -> (0, 1=w257:i16)
            n142 = Equal To 0?(x=w257) -> (x = 0?=w256:bool)
            n143 = case shown="True" w256 {
              tunnel: [TRUE ("T button?") w260] -> w251
              frame False {
              }
              frame True {
                # "Log Data Check"
                n144 = Two Button Dialog(message="You are not currently logging data!\nDo you wish to continue?", 1:"No" ("T button name (\"OK\")"), 2:"Yes" ("T button name (\"OK\")")) -> (T button?=w260:bool)
              }
            }
            n145 = Equal?(x=2.0, y=2.0) -> (x = y?=w252:bool)
            n146 = And(x=w252, y=w251) -> (x .and. y?=w253:bool)
            n147 = case shown="True" w253 {
              frame False {
              }
              frame True {
                n148 = flat-sequence {
                  tunnel: "Cycle size" -> [w287]
                  tunnel: [w287] -> w276
                  tunnel: [w290] -> w285
                  tunnel: w276 -> [w290]
                  tunnel: w285 -> [w293]
                  tunnel: [w293] -> w284
                  tunnel: w284 -> [w296]
                  tunnel: [w296] -> w283
                  tunnel: w283 -> [w299]
                  tunnel: [w299] -> w275
                  tunnel: w275 -> [w302]
                  tunnel: [w302] -> w274
                  tunnel: [w305] -> w286
                  tunnel: w274 -> [w305]
                  tunnel: [w308] -> w282
                  tunnel: w286 -> [w308]
                  tunnel: w282 -> [w311]
                  tunnel: [w311] -> w280
                  tunnel: w280 -> [w314]
                  tunnel: [w314] -> w279
                  tunnel: w279 -> [w317]
                  tunnel: [w317] -> w278
                  tunnel: w278 -> [w323]
                  tunnel: [w323] -> w277
                  tunnel: w277 -> [w334]
                  frame #0 {
                    n149 = call-poly <vilib>:"Read From Spreadsheet File.vi"() -> ("all rows"=w288:dbl[][])  [unwired: 7 in, 4 out]
                    n150 = Reshape Array(w288, w287) -> (→"CO":dbl[])
                  }
                  frame #1 {
                    n151 = call-poly <vilib>:"Read From Spreadsheet File.vi"() -> ("all rows"=w292:dbl[][])  [unwired: 7 in, 4 out]
                    n152 = Reshape Array(w292, w290) -> (→"Air Cyc 1":dbl[])
                  }
                  frame #2 {
                    n153 = call-poly <vilib>:"Read From Spreadsheet File.vi"() -> ("all rows"=w294:dbl[][])  [unwired: 7 in, 4 out]
                    n154 = Reshape Array(w294, w293) -> (→"Air Cyc 2":dbl[])
                  }
                  frame #3 {
                    n155 = call-poly <vilib>:"Read From Spreadsheet File.vi"() -> ("all rows"=w298:dbl[][])  [unwired: 7 in, 4 out]
                    n156 = Reshape Array(w298, w296) -> (→"HC Cyc 1":dbl[])
                  }
                  frame #4 {
                    n157 = call-poly <vilib>:"Read From Spreadsheet File.vi"() -> ("all rows"=w301:dbl[][])  [unwired: 7 in, 4 out]
                    n158 = Reshape Array(w301, w299) -> (→"HC Cyc 2":dbl[])
                  }
                  frame #5 {
                    n159 = call-poly <vilib>:"Read From Spreadsheet File.vi"() -> ("all rows"=w303:dbl[][])  [unwired: 7 in, 4 out]
                    n160 = Reshape Array(w303, w302) -> (→"NO":dbl[])
                  }
                  frame #6 {
                    n161 = call-poly <vilib>:"Read From Spreadsheet File.vi"() -> ("all rows"=w306:dbl[][])  [unwired: 7 in, 4 out]
                    n162 = Reshape Array(w306, w305) -> (→"Air Bal":dbl[])
                  }
                  frame #7 {
                    n163 = call-poly <vilib>:"Read From Spreadsheet File.vi"() -> ("all rows"=w310:dbl[][])  [unwired: 7 in, 4 out]
                    n164 = Reshape Array(w310, w308) -> (→"HC Bal":dbl[])
                  }
                  frame #8 {
                    n165 = call-poly <vilib>:"Read From Spreadsheet File.vi"() -> ("all rows"=w312:dbl[][])  [unwired: 7 in, 4 out]
                    n166 = Reshape Array(w312, w311) -> (→"SO Valve 1":dbl[])
                  }
                  frame #9 {
                    n167 = call-poly <vilib>:"Read From Spreadsheet File.vi"() -> ("all rows"=w315:dbl[][])  [unwired: 7 in, 4 out]
                    n168 = Reshape Array(w315, w314) -> (→"SO Valve 2":dbl[])
                  }
                  frame #10 {
                    n169 = call-poly <vilib>:"Read From Spreadsheet File.vi"() -> ("all rows"=w319:dbl[][])  [unwired: 7 in, 4 out]
                    n170 = Reshape Array(w319, w317) -> (→"Open/Closed \nLoop":dbl[])
                  }
                  frame #11 {
                    n171 = local read "Open/Closed \nLoop"() -> (w324:dbl[])
                    n172 = local read "SO Valve 1"() -> (w326:dbl[])
                    n173 = local read "SO Valve 2"() -> (w325:dbl[])
                    n174 = local read "HC Cyc 2"() -> (w329:dbl[])
                    n175 = local read "HC Cyc 1"() -> (w328:dbl[])
                    n176 = local read "Air Cyc 1"() -> (w322:dbl[])
                    n177 = local read "Air Cyc 2"() -> (w327:dbl[])
                    n178 = local read "HC Bal"() -> (w331:dbl[])
                    n179 = local read "Air Bal"() -> (w330:dbl[])
                    n180 = local read "NO"() -> (w320:dbl[])
                    n181 = local read "CO"() -> (w321:dbl[])
                    n182 = Build Array (concatenate)(w323, w321, w322, w327, w328, w329, w320, w330, w331, w326, w325, w324) -> (w332:dbl[])
                    n183 = shared-variable "RT CompactRIO Target 2\\Library 1.lvlib\\Inject_Arrays"(w332) -> ()  [unwired: 1 in, 1 out]
                  }
                  frame #12 {
                    n184 = call-poly <vilib>:"Read From Spreadsheet File.vi"() -> ("all rows"=w335:dbl[][])  [unwired: 7 in, 4 out]
                    n185 = Reshape Array(w335, w334) -> (w333:dbl[])
                    "Lambda" <- w333
                    n186 = shared-variable "RT CompactRIO Target 2\\Library 1.lvlib\\Inject_Arrays_Lambda"(w333) -> ()  [unwired: 1 in, 1 out]
                  }
                }
              }
            }
            n187 = case shown="True" w251 {
              tunnel: w258 -> [_ w265]
              frame False {
              }
              frame True {
                n188 = flat-sequence {
                  tunnel: w265 -> [w268]
                  tunnel: [w268] -> w264
                  tunnel: w264 -> [w272]
                  frame #0 {
                    n189 = local write "Enum 1"(u16 1 ("Test number")) -> ()
                    "Test number" <- "Select Test Type"
                  }
                  frame #1 {
                    n190 = Enqueue Element(queue=w272, element=Control_3."main" ("Enum")) -> (queue out=w270:refnum<queue>)  [unwired: 2 in, 2 out]
                    n191 = property on="Stop Test" class="Bool (strict)"("DisabledEnum"=T11."Enabled" ("Disabled")) -> ()  [unwired: 2 in, 2 out]
                    n192 = Enqueue Element(queue=w270, element=Control_3."start test" ("Enum")) -> ()  [unwired: 2 in, 3 out]
                  }
                }
              }
            }
          }
        }
      }
      event "Log Test Data": Value Change {
        n193 = event-data() -> ()  [unwired: 1 in, 6 out]
        n194 = property on="File Name" class="Str (strict)"() -> ("Value"=w338:T5)  [unwired: 2 in, 2 out]
        n195 = String Length(string=w338) -> (length=w337:i32)
        n196 = Equal To 0?(x=w337) -> (x = 0?=w336:bool)
        n197 = case shown="True" w336 {
          frame False {
          }
          frame True {
            n198 = One Button Dialog(message="A filename has not been entered!") -> ()  [unwired: 1 in, 1 out]
          }
        }
      }
      event "Stop Test": Value Change {
        n199 = event-data() -> ()  [unwired: 1 in, 6 out]
        n200 = case shown="True" "Stop Test" {
          tunnel: w341 -> [_ w343]
          frame False {
          }
          frame True {
            n201 = flat-sequence {
              tunnel: w343 -> [w349]
              tunnel: [w349] -> w347
              tunnel: [w348] -> w346
              tunnel: w347 -> [w353]
              tunnel: [w352] -> w345
              tunnel: w346 -> [w352]
              tunnel: [w351] -> w344
              tunnel: w345 -> [w357]
              tunnel: w344 -> [w356]
              tunnel: [T11."Disabled and Grayed Out" ("Disabled")] -> _
              frame #0 {
                n202 = local read "Connected?"() -> (w348:bool)
                n203 = local write "Stop Cmd"(T1 1.0 ("Stop Cmd")) -> ()
              }
              frame #1 {
                n204 = Enqueue Element(queue=w353, element=Control_3."main" ("Enum")) -> (queue out=w351:refnum<queue>)  [unwired: 2 in, 2 out]
              }
              frame #2 {
                n205 = case shown="True" w357 {
                  tunnel: w356 -> [w358 w361]
                  tunnel: [w358 w360] -> _
                  frame False {
                  }
                  frame True {
                    n206 = local write "Connected?"(FALSE ("Connected?")) -> ()
                    n207 = Enqueue Element(queue=w361, element=Control_3."Multigas disconnect" ("Enum")) -> (queue out=w360:refnum<queue>)  [unwired: 2 in, 2 out]
                  }
                }
              }
            }
            n208 = local write "Start Test"(FALSE ("Start Test")) -> ()
          }
        }
      }
      event "Stopped?": Value Change {
        n209 = event-data() -> ()  [unwired: 1 in, 5 out]
        n210 = flat-sequence {
          tunnel: w365 -> [w369]
          tunnel: [w368] -> w364
          tunnel: [w367] -> w363
          tunnel: w364 -> [w371]
          tunnel: w363 -> [w370]
          frame #0 {
            n211 = local read "Connected?"() -> (w367:bool)
            n212 = Enqueue Element(queue=w369, element=Control_3."main" ("Enum")) -> (queue out=w368:refnum<queue>)  [unwired: 2 in, 2 out]
          }
          frame #1 {
            n213 = case shown="True" w370 {
              tunnel: w371 -> [_ w372]
              frame False {
              }
              frame True {
                n214 = local write "Connected?"(FALSE ("Connected?")) -> ()
                n215 = Enqueue Element(queue=w372, element=Control_3."Multigas disconnect" ("Enum")) -> ()  [unwired: 2 in, 3 out]
              }
            }
          }
        }
      }
      event "Alarm ack": Value Change {
        # "system alarm - set to off"
        n216 = event-data() -> ()  [unwired: 1 in, 5 out]
        n217 = local write "Acknowledge"(TRUE ("Acknowledge")) -> ()
        n218 = property on="Soft Alarm" class="Bool (strict)"("Value"=FALSE ("Acknowledge")) -> ()  [unwired: 2 in, 2 out]
        n219 = property on="Alarm ack" class="Bool"("DisabledEnum"=T11."Disabled and Grayed Out" ("Disabled")) -> ()  [unwired: 2 in, 2 out]
      }
      event "Purge System": Value Change {
        n220 = event-data() -> ()  [unwired: 1 in, 5 out]
        n221 = flat-sequence {
          tunnel: w379 -> [w381]
          tunnel: [w381] -> w378
          tunnel: w378 -> [w382]
          frame #0 {
            n222 = local write "Enum 1"(u16 4 ("Test number")) -> ()
          }
          frame #1 {
            n223 = Enqueue Element(queue=w382, element=Control_3."start test" ("Enum")) -> ()  [unwired: 2 in, 3 out]
          }
        }
      }
      event "Clear log": Value Change {
        n224 = event-data() -> ()  [unwired: 1 in, 5 out]
        n225 = local write "Table"(string[][] [] ("Table")) -> ()
      }
      event "Adv Settings": Value Change {
        # "To be updated"
        # "SO2 conc\nNOx conc\nCO conc\nHC conc\nBleed ratio N2\nBleed ratio CO2"
        n226 = event-data() -> ()  [unwired: 1 in, 6 out]
        n227 = call "Advanced settings MAX.vi"() -> ("output cluster"=→"output cluster":T2)  [unwired: 1 in]
      }
      event "Home": Value Change {
        w387 = FALSE
        n228 = event-data() -> ()  [unwired: 1 in, 6 out]
      }
      event "Performance": Value Change {
        w390 = FALSE
        n229 = event-data() -> ()  [unwired: 1 in, 6 out]
      }
      event "Ageing": Value Change {
        w394 = FALSE
        n230 = event-data() -> ()  [unwired: 1 in, 6 out]
      }
      event "System": Value Change {
        w398 = FALSE
        n231 = event-data() -> ()  [unwired: 1 in, 6 out]
      }
      event "MFC": Value Change {
        w402 = FALSE
        n232 = event-data() -> ()  [unwired: 1 in, 6 out]
      }
      event "Analyser": Value Change {
        w407 = FALSE
        n233 = event-data() -> ()  [unwired: 1 in, 6 out]
      }
      event "Alarm": Value Change {
        w410 = FALSE
        n234 = event-data() -> ()  [unwired: 1 in, 6 out]
      }
    }
    "stop 2" <- w68
    n235 = local write "Tab Control"(w66) -> ()
    n236 = case shown="False" w65 {
      tunnel: [w80 w88] -> w67
      tunnel: w66 -> [w80 _]
      tunnel: w64 -> [_ w88]
      tunnel: w63 -> [_ w87]
      tunnel: w62 -> [_ w86]
      tunnel: w61 -> [_ w85]
      tunnel: w60 -> [_ w84]
      tunnel: w59 -> [_ w83]
      tunnel: w58 -> [_ w82]
      tunnel: w57 -> [_ w81]
      tunnel: [w78 w87] -> w56
      tunnel: [w77 w86] -> w55
      tunnel: [w73 w85] -> w54
      tunnel: [w74 w84] -> w53
      tunnel: [w75 w83] -> w52
      tunnel: [w76 w82] -> w51
      tunnel: [w79 w81] -> w50
      tunnel: w49 -> [w78 _]
      tunnel: w48 -> [w77 _]
      tunnel: w47 -> [w79 _]
      tunnel: w46 -> [w76 _]
      tunnel: w45 -> [w75 _]
      tunnel: w44 -> [w74 _]
      tunnel: w43 -> [w73 _]
      frame False {
      }
      frame True {
      }
    }
    n237 = local write "MFC"(w52) -> ()
    n238 = local write "Home"(w56) -> ()
    n239 = local write "System"(w53) -> ()
    n240 = local write "Alarm"(w50) -> ()
    n241 = local write "Ageing"(w54) -> ()
    n242 = local write "Analyser"(w51) -> ()
    n243 = local write "Performance"(w55) -> ()
  }
  n244 = node-c288(nitl_modes."Discard missed periods, maintain original phase" ("Mode")) -> (w14:T12)  [unwired: 4 in]
  n245 = node-c288() -> (w7:T12)  [unwired: 4 in]
  n246 = timed-loop {
    timing: w14 -> [_]
    timing-out: [_] -> w13
    shift-right: [w539] -> _
    shift-left: path "" -> [w505]
    shift-right: [w598] -> _
    shift-left: w8 -> [w633]
    shift-right: [w540] -> _
    shift-left: _ -> [w608]
    shift-right: [w588] -> _
    shift-left: w8 -> [w591]
    shift-right: [w589] -> _
    shift-left: w8 -> [w590]
    shift-right: [w531] -> _
    shift-left: 0 ("t") -> [w530]
    shift-right: [w521] -> _
    shift-left: _ -> [w510]
    shift-right: [w520] -> _
    shift-left: _ -> [w511]
    shift-right: [w519] -> _
    shift-left: _ -> [w512]
    shift-right: [w518] -> _
    shift-left: _ -> [w513]
    shift-right: [w517] -> _
    shift-left: _ -> [w514]
    shift-right: [w516] -> _
    shift-left: _ -> [w515]
    shift-right: [w495] -> _
    shift-left: _ -> [w496]
    stop <- w632 stop-if-true
    w547 = 54321.0 ("y")
    # "Flow Rate Guide"
    # "Temperature Guide"
    # "0   Flow Rate 1\n1   Flow Rate 2\n     ECM 1\n     ECM 2\n2   CO2 U\n3   CO U\n4   HC U\n5   O2 U\n7   CO2 D\n8   CO D\n9   HC D\n10 O2 D\n12 TC1X\n13 TC2A\n14 TC3Y\n15 TC4B\n16 TC5\n17 TC6\n32 Venturi 1\n33 Venturi 2\n34 Tank\n35 Bearing 1\n36 Bearing 2\n38 Ex A\n39 Ex B\n40 Ex C\n41 Ex D\n     MFC Box\n42 Furnace 1\n43 Furnace 2\n44 NO 1 ?? \n45 Lambda 1\n46 NO 2 ??\n47 Lambda 2"
    n247 = node-c288() -> (→"Finished Late? [i-1]":bool, →"Iteration Duration":i64)  [unwired: 1 in, 1 out]
    n248 = shared-variable "RT CompactRIO Target 2\\Library 1.lvlib\\DATA"() -> (w631:dbl[])  [unwired: 1 in, 1 out]
    n249 = local read "MKS"() -> (w426:bool)
    n250 = Type Cast(type=w631, x=w631) -> (*(type *) &x=w641:dbl[])
    n251 = local read "Advanced Logging"() -> (w544:bool)
    n252 = Delete From Array(array=w641, length=4, index=0) -> (deleted portion=w638:dbl[], array with subset deleted=w421:dbl[])
    n253 = call "MKS.vi"("IP Address"="192.168.254.1", "Connect"=w426) -> ("Emissions"=w508:dbl[])  [unwired: 9 in]
    n254 = call "MKS.vi"("IP Address"="192.168.254.2", "Connect"=FALSE) -> ("Emissions"=w509:dbl[])  [unwired: 9 in]
    n255 = local read "Full system?"() -> (w538:bool)
    n256 = Index Array(array=w508, index=0) -> (element=w551:dbl)
    n257 = Index Array(array=w509, index=0) -> (element=w549:dbl)
    n258 = case shown="True" w544 {
      tunnel: [w738 w789] -> w545
      tunnel: w421 -> [w739 w789]
      tunnel: [w737 "Time\tFlow 1 g/s\tFlow 2 g/s\tECM 1\tECM 2\tTank Pressure\tTC1X\tTC2A\tTCY\tTC4B\tTC5\tTC6\tTC7\tTC8\tTC9\tTC10\tTC11\tTC12\tTC13\tTC14\tTC15\tTC16\tTC17\tTC18\tTC19\tTC20\tC Vent 1\tTC Vent 2\tTC Tank\tTC Fan B1\tTC Fan B2\tTC Cab\tTC Ex A\tTC Ex B\tTC Ex C\tTC Ex D\tSpare\tTC Furn 1\tTC Furn 2\tRapidox\tCO2 U %\tCO U %\tHC U ppm\tO2 U %\tNO U ppm\tCO2 D %\tCO D %\tHC D ppm\tO2 D %\tNO D ppm\tSwitch\tUEGO 1\tUEGO 2\tUEGO 3\tUEGO 4\tNOx Can 1\tNOx Can 2" ("Heading string 2")] -> w543
      tunnel: w538 -> [w736 _]
      frame False {
        n259 = case shown="True" w736 {
          tunnel: w739 -> [w754 w769]
          tunnel: [w745 w771] -> w738
          tunnel: ["Time\tFlow 1 g/s\tCO2 U %\tCO U %\tHC U ppm\tO2 U %\tNO U ppm\tCO2 D %\tCO D %\tHC D ppm\tO2 D %\tNO D ppm\tTC1X\tTC2A\tTCY\tTC4B\tTC5\tTC6\tTC7\tTC8\tRapidox\tLambda 1\tLambda 2\tNOX 1 ppm\tNOX 2 ppm\tUEGO 1\tUEGO 2" ("Heading string 2") "Time\tFlow 1 g/s\tFlow 2 g/s\tCO2 U %\tCO U %\tHC U ppm\tO2 U %\tNO U ppm\tCO2 D %\tCO D %\tHC D ppm\tO2 D %\tNO D ppm\tTC1X\tTC2A\tTCY\tTC4B\tTC5\tTC6\tTC7\tTC8\tRapidox\tLambda 1\tLambda 2\tNOX 1 ppm\tNOX 2 ppm\tUEGO 1\tUEGO 2" ("Heading string 2")] -> w737
          frame False {
            n260 = Delete From Array(array=w754, length=21, index=0) -> (deleted portion=w741:dbl[], array with subset deleted=w753:dbl[])
            n261 = Index Array(array=w753, index #1=47 ("index"), index #2=48 ("index"), index #3=49 ("index"), index #4=50 ("index"), index #5=51 ("index"), index #6=52 ("index"), index #7=53 ("index")) -> (element #1=w752:dbl, element #2=w751:dbl, element #3=w750:dbl, element #4=w749:dbl, element #5=w748:dbl, element #6=w747:dbl, element #7=w746:dbl)
            n262 = Delete From Array(array=w741, length=1, index=2) -> (array with subset deleted=w740:dbl[])  [unwired: 1 out]
            n263 = Build Array (concatenate)(w740, w752, w751, w750, w749, w748, w747, w746) -> (w745:dbl[])
          }
          frame True {
            n264 = Delete From Array(array=w769, length=21, index=0) -> (deleted portion=w766:dbl[], array with subset deleted=w770:dbl[])
            n265 = Index Array(array=w770, index #1=47 ("index"), index #2=48 ("index"), index #3=49 ("index"), index #4=50 ("index"), index #5=51 ("index"), index #6=52 ("index"), index #7=53 ("index")) -> (element #1=w778:dbl, element #2=w777:dbl, element #3=w776:dbl, element #4=w775:dbl, element #5=w774:dbl, element #6=w773:dbl, element #7=w772:dbl)
            n266 = Delete From Array(array=w766, length=2, index=1) -> (array with subset deleted=w764:dbl[])  [unwired: 1 out]
            n267 = Build Array (concatenate)(w764, w778, w777, w776, w775, w774, w773, w772) -> (w771:dbl[])
          }
        }
      }
      frame True {
        (unwired) "Time\tFlow 1 g/s\tFlow 2 g/s\tECM AFR\tCO2 U %\tCO U %\tHC U ppm\tO2 U %\tNO U ppm\tCO2 D %\tCO D %\tHC D ppm\tO2 D %\tNO D ppm\tTC1X\tTC2A\tTCY\tTC4B\tTC5\tTC6\tTC7\tTC8\tTC9\tTC10\tTC11\tTC12\tTC13\tTC14\tTC15\tTC16\tTC17\tTC18\tTC19\tTC20\tTC Vent 1\tTC Vent 2\tTC Fan B1\tTC Fan B2\tTC Cab\tTC Ex A\tTC Ex B\tTC Ex C\tTC Ex D\tTC Furn 1\tTC Furn 2\tNOX 1 ppm\tNLambda 1\tNOX 2 ppm\tNLambda 2\tEGO 1\tEGO 2\tEGO 3\tEGO 4\tCO2 U %\tCO U %\tHC U ppm\tO2 U %\tNO U ppm\tCO2 D %\tCO D %\tHC D ppm\tO2 D %\tNO D ppm\r\n" ("Heading string 2")
      }
    }
    n268 = Not Equal?(x=w551, y=w547) -> (x != y?=w550:bool)
    n269 = Not Equal?(x=w547, y=w549) -> (x != y?=w548:bool)
    n270 = Index Array(array=w638) -> (element #1=w540:dbl, element #2=w611:dbl, element #3=w424:dbl, element #4=w607:dbl)  [unwired: 4 in]
    "Error" <- w424
    n271 = case shown="False" w550 {
      tunnel: [w795 w806] -> w506
      tunnel: w509 -> [w794 w805]
      tunnel: w508 -> [_ w804]
      tunnel: w548 -> [w793 w803]
      tunnel: [w792 w800] -> w546
      frame False {
        n272 = case shown="False" w793 {
          tunnel: [dbl[] [54321.0] w799] -> w795
          tunnel: w794 -> [_ w799]
          tunnel: ["\r\n" ("Heading string 2") "\tNO\tNO2 (150)\tNO2 (2000)\tN2O\tNH3 (300)\tNH3 (3000)\tHNCO (400)\tH2O\tCO2\tCO (500)\tCO (1)\tCH4 (250)\tCH4 (3000)\tNOxP\tPropane\r\n" ("Heading string 2")] -> w790
          frame False {
          }
          frame True {
          }
        }
        n273 = Build Array(" " ("Heading string 2"), w790) -> (w792:string[])
      }
      frame True {
        n274 = case shown="True" w803 {
          tunnel: [w808 w812] -> w806
          tunnel: w805 -> [_ w811]
          tunnel: w804 -> [w808 w810]
          tunnel: ["\rn" ("Heading string 2") "\tNO\tNO2 (150)\tNO2 (2000)\tN2O\tNH3 (300)\tNH3 (3000)\tHNCO (400)\tH2O\tCO2\tCO (500)\tCO (1)\tCH4 (250)\tCH4 (3000)\tNOxP\tPropane\r" ("Heading string 2")] -> w801
          frame False {
          }
          frame True {
            n275 = Build Array (concatenate)(w810, w811) -> (w812:dbl[])
          }
        }
        n276 = Build Array("\tNO\tNO2 (150)\tNO2 (2000)\tN2O\tNH3 (300)\tNH3 (3000)\tHNCO (400)\tH2O\tCO2\tCO (500)\tCO (1)\tCH4 (250)\tCH4 (3000)\tNOxP\tPropane" ("Heading string 2"), w801) -> (w800:string[])
      }
    }
    n277 = To Unsigned Long Integer(number=w607) -> (unsigned 32bit integer=w606:u32)
    n278 = Number To Boolean Array(number=w606) -> (Boolean array=w621:bool[])
    n279 = Index Array(array=w621) -> (element #2=w619:bool, element #3=w618:bool, element #4=w603:bool, element #5=→"ExtAnUp":bool, element #6=→"ExtAnDn":bool)  [unwired: 6 in, 1 out]
    "Extractor Fan On" <- w603
    n280 = local read "7170"() -> (w414:bool)
    n281 = case shown="0, Default" w611 {
      tunnel: [w832 TRUE FALSE] -> w610
      tunnel: [w833 FALSE TRUE] -> w609
      frame 0, Default {
        n282 = local read "Pass"() -> (w833:bool)
        n283 = local read "Fail"() -> (w832:bool)
      }
      frame 1 {
      }
      frame 2 {
      }
    }
    "Pass" <- w609
    "Fail" <- w610
    n284 = Or(x=w619, y=w618) -> (x .or. y?=→"Doors Open":bool)
    n285 = Not(x=w603) -> (.not. x?=→"Doors Unlocked":bool)
    n286 = Less?(x=w540, y=w608) -> (x < y?=w605:bool)
    n287 = Path To String(path="File Path") -> (string=w601:string)
    n288 = local read "Connected"() -> (w604:bool)
    n289 = Concatenate Strings(w601, "\\" ("string"), "File Name") -> (w554:string)
    n290 = call "Mexa_7170.vi"("String 1 In"=w514, "Connect"=w414, "connection ID 1 In"=w513, "error out 1 In"=w512, "connection ID 2 In"=w511, "error out 2 In"=w510, "Time In"=w515) -> ("Emissions"=w507:dbl[], "String 1 Out"=w517:string, "connection ID 1 Out"=w518:refnum<k5>, "error 1 out"=w519:errorcluster, "connection ID 2 Out"=w520:refnum<k16>, "Time Out"=w516:i16, "error 2 out"=w521:errorcluster)  [unwired: 2 in]
    "Emissions" <- w507
    n291 = Build Array (concatenate)(w507, w506) -> (w419:dbl[])
    n292 = And(x=w604, y=w605) -> (x .and. y?=w597:bool)
    n293 = Build Array (concatenate)(w421, w419) -> (w420:dbl[])
    n294 = local write "Stopped?"(w597) -> ()
    n295 = Equal To 0?(x=w424) -> (x = 0?=w542:bool)
    n296 = Equal To 0?(x=w540) -> (x = 0?=w541:bool)
    n297 = Build Array (concatenate)(w545, w419) -> (w634:dbl[])
    n298 = Equal?(x=w540, y=2.0) -> (x = y?=w562:bool)
    n299 = String To Path(string=w554) -> (path=w599:path)
    n300 = Build Array(w542, w541) -> (w616:bool[])
    n301 = Equal?(x=w540, y=3.0) -> (x = y?=w559:bool)
    n302 = Equal?(x=w540, y=4.0) -> (x = y?=w557:bool)
    n303 = Boolean Array To Number(Boolean array=w616) -> (number=w615:u32)
    n304 = Index Array(array=w420, index=4) -> (element=→"Pressure":dbl)
    n305 = Not Equal?(x=w599, y=w505) -> (x != y?=w643:bool)
    n306 = Compound Arithmetic op=OR(w562, w559, w557) -> (w561:bool)
    n307 = case shown="3" w615 {
      tunnel: [w858 w859 w864 w866] -> _
      tunnel: [w858 w859 w864 w866] -> w614
      tunnel: [w858 w859 w864 w866] -> w613
      tunnel: [w858 w859 w862 w866] -> w612
      tunnel: [T11."Enabled" ("Disabled") T11."Enabled" ("Disabled") w862 w866] -> _
      tunnel: [FALSE FALSE FALSE TRUE] -> w596
      frame 0, Default {
        w858 = T11."Disabled and Grayed Out" ("Disabled")
      }
      frame 1 {
        w859 = T11."Disabled and Grayed Out" ("Disabled")
      }
      frame 2 {
        w862 = T11."Enabled" ("Disabled")
        w864 = T11."Disabled and Grayed Out" ("Disabled")
      }
      frame 3 {
        w866 = T11."Enabled" ("Disabled")
        (unwired) T11."Disabled and Grayed Out" ("Disabled")
      }
    }
    n308 = local read "Log Test Data"() -> (w555:bool)
    n309 = for {
      tunnel: w634 -> [w874] mode=indexing
      tunnel: [w873] -> w645 mode=indexing
      n310 = Number To Fractional String(number=w874, precision (6)=i16 3) -> (F-format string=w873:string)  [unwired: 2 in]
    }
    n311 = Select(t=w599, s=w643, f=w505) -> (s? t:f=w644:path)
    n312 = And(x=w555, y=w561) -> (x .and. y?=w660:bool)
    "Log?" <- w660
    n313 = case shown="True" w643 {
      tunnel: w644 -> [w867 w872]
      tunnel: [w867 w871] -> w642
      tunnel: w546 -> [_ w869]
      tunnel: w543 -> [_ w868]
      frame False {
      }
      frame True {
        # "setting up the header"
        n314 = Build Array (concatenate)(w868, w869) -> (w870:string[])
        n315 = call-poly <vilib>:"Write To Spreadsheet File.vi"("1D data"=w870, "file path (dialog if empty)"=w872) -> ("new file path (Not A Path if cancelled)"=w871:path)  [unwired: 6 in]
      }
    }
    n316 = Equal?(x=w540, y=0.0) -> (x = y?=w585:bool)
    n317 = case shown="0, Default" w540 {
      tunnel: [w819 w821 w824 w825 TRUE FALSE] -> w435
      tunnel: [w819 w821 w824 TRUE w827 w830] -> w433
      tunnel: [TRUE w821 w824 w825 w827 w830] -> w432
      tunnel: [w819 TRUE TRUE w825 w827 w830] -> w416
      frame 0, Default {
        w819 = FALSE
      }
      frame 1 {
        w821 = FALSE
      }
      frame 2 {
        w824 = FALSE
      }
      frame 3 {
        w825 = FALSE
      }
      frame 4 {
        w827 = FALSE
        n318 = local write "Stop Cmd"(T1 0.0 ("Stop Cmd")) -> ()
      }
      frame 5 {
        w830 = FALSE
      }
    }
    n319 = property on="Execute Leak Test Button" class="Bool"("DisabledEnum"=w614) -> ()  [unwired: 2 in, 2 out]
    n320 = property on="Compile Test Button" class="Bool"("DisabledEnum"=w613) -> ()  [unwired: 2 in, 2 out]
    n321 = property on="Purge System" class="Bool"("DisabledEnum"=w612) -> ()  [unwired: 2 in, 2 out]
    n322 = property class="VI"("Front Panel.Closeable"=w596) -> ()  [unwired: 2 in, 2 out]
    n323 = local read "Full system?"() -> (w586:bool)
    n324 = Index Array(array=w419, index #1=0 ("index"), index #2=1 ("index"), index #3=2 ("index"), index #4=3 ("index")) -> ()  [unwired: 4 out]
    n325 = Equal?(x=w424, y=1024.0) -> (x = y?=w422:bool)
    n326 = case shown="True" "Demo On" {
      tunnel: w435 -> [w664 w668]
      tunnel: [w664 w667] -> w434
      tunnel: w433 -> [w666 _]
      tunnel: w432 -> [w665 _]
      tunnel: [w665 w667] -> w431
      tunnel: [w666 TRUE] -> w430
      tunnel: [w664 w668] -> w418
      tunnel: [w663 w667] -> w417
      tunnel: w416 -> [w663 _]
      frame False {
      }
      frame True {
        w667 = FALSE
      }
    }
    "Cool Down" <- w434
    "Test In Progress" <- w430
    "Standby" <- w431
    "Warm Up" <- w417
    n327 = case shown="True" w422 {
      tunnel: w424 -> [w661 _]
      tunnel: [w661 0.0 ("Numeric")] -> w425
      frame False {
      }
      frame True {
      }
    }
    n328 = Build Array(w586, w585) -> (w587:bool[])
    n329 = local write "Stop Test"(w418) -> ()
    n330 = Boolean Array To Number(Boolean array=w587) -> (number=w584:u32)
    n331 = call "Demo_Guide.vi"("Time In"=w496, "Temperature Sync"="Demo Sync", "Duration -1"="Duration -1", "TempGuide"="Demo On") -> ("Output array"=w471:dbl[], "Time out"=w495:i32)  [unwired: 6 in]
    n332 = Not Equal To 0?(x=w425) -> (x != 0?=w636:bool)
    n333 = Not Equal?(x=w425, y=w633) -> (x != y?=w635:bool)
    n334 = case shown="True" w660 {
      tunnel: w642 -> [w878 w886]
      tunnel: [w878 w898] -> w539
      tunnel: w645 -> [_ w894]
      tunnel: w591 -> [_ w887]
      tunnel: w590 -> [w877 w882]
      tunnel: [w877 w884] -> w589
      tunnel: [w876 w883] -> w588
      frame False {
        n335 = local read "Log interval (seconds)"() -> (w876:T1)
      }
      frame True {
        n336 = Get Date/Time In Seconds() -> (seconds since 1Jan1904=w895:timestamp)
        n337 = Decrement(x=w887) -> (x-1=w888:T1)
        n338 = Less Than 0?(x=w888) -> (x < 0?=w889:bool)
        n339 = Equal To 0?(x=w888) -> (x = 0?=w890:bool)
        n340 = Build Array(w889, w890) -> (w891:bool[])
        n341 = Path To String(path=w886) -> (string=w881:string)
        "File name" <- w881
        n342 = Format Date/Time String(time format string (%c)="%d/%m/%y %H:%M:%S", seconds (now)=w895) -> (date/time string=w896:string)  [unwired: 1 in]
        n343 = Boolean Array To Number(Boolean array=w891) -> (number=w892:u32)
        n344 = case shown="2" w892 {
          tunnel: w887 -> [w905 w906 _]
          tunnel: [w904 w906 w909] -> w883
          tunnel: w881 -> [w903 w908 w912]
          tunnel: [w900 w908 w910] -> w885
          tunnel: [w899 w907 w911] -> w884
          tunnel: w882 -> [w899 w907 w915]
          frame 0, Default {
            n345 = Number To Decimal String(number=w899) -> (decimal integer string=w901:string)  [unwired: 1 in]
            n346 = call <vilib>:"Space Constant.vi"() -> ("String"=w902:string)
            n347 = Decrement(x=w905) -> (x-1=w904:T1)
            n348 = Concatenate Strings(w903, w902, w901) -> (w900:string)
          }
          frame 1 {
          }
          frame 2 {
            n349 = Increment(x=w915) -> (x+1=w911:dbl)
            n350 = local read "Log interval (seconds)"() -> (w909:T1)
            n351 = Number To Decimal String(number=w911) -> (decimal integer string=w913:string)  [unwired: 1 in]
            n352 = call <vilib>:"Space Constant.vi"() -> ("String"=w914:string)
            n353 = Concatenate Strings(w912, w914, w913) -> (w910:string)
          }
        }
        n354 = Build Array (concatenate)(w896, w894) -> (w880:string[])
        n355 = String To Path(string=w885) -> (path=w879:path)
        n356 = call-poly <vilib>:"Write To Spreadsheet File.vi"("append to file? (new file:F)"=TRUE, "1D data"=w880, "file path (dialog if empty)"=w879) -> ("new file path (Not A Path if cancelled)"=w898:path)  [unwired: 5 in]
      }
    }
    n357 = And(x=w636, y=w635) -> (x .and. y?=w637:bool)
    n358 = Index Array(array=w420, index #1=0 ("index"), index #2=1 ("index"), index #3=58 ("index"), index #4=55 ("index"), index #5=42 ("index"), index #6=44 ("index"), index #7=45 ("index"), index #8=47 ("index"), index #9=60 ("index"), index #10=46 ("index"), index #11=5 ("index"), index #12=6 ("index"), index #13=7 ("index"), index #14=8 ("index"), index #15=9 ("index"), index #16=10 ("index"), index #17=25 ("index"), index #18=26 ("index"), index #19=27 ("index"), index #20=28 ("index"), index #21=29 ("index"), index #22=31 ("index"), index #23=32 ("index"), index #24=33 ("index"), index #25=34 ("index"), index #26=36 ("index"), index #27=37 ("index"), index #28=43 ("index"), index #29=48 ("index"), index #30=45 ("index"), index #31=46 ("index"), index #32=2 ("index"), index #33=3 ("index")) -> (element #1=w533:dbl, element #2=w532:dbl, element #3=w494:dbl, element #4=w492:dbl, element #5=w490:dbl, element #6=w489:dbl, element #7=w488:dbl, element #8=w487:dbl, element #9=w486:dbl, element #10=w484:dbl, element #11=w483:dbl, element #12=w481:dbl, element #13=w479:dbl, element #14=w477:dbl, element #15=w475:dbl, element #16=w473:dbl, element #17=w466:dbl, element #18=w464:dbl, element #19=w462:dbl, element #20=w460:dbl, element #21=w458:dbl, element #22=w456:dbl, element #23=w454:dbl, element #24=w452:dbl, element #25=w450:dbl, element #26=→"Furnace temp 1":dbl, element #27=→"Furnace temp 2":dbl, element #28=w448:dbl, element #29=w446:dbl, element #30=w444:dbl, element #31=w442:dbl, element #32=w440:dbl, element #33=w438:dbl)
    n359 = case shown="False" w637 {
      tunnel: w425 -> [w839 w851]
      tunnel: w635 -> [w842 _]
      tunnel: [w838 w851] -> w598
      frame False {
        n360 = Equal To 0?(x=w839) -> (x = 0?=w843:bool)
        n361 = And(x=w843, y=w842) -> (x .and. y?=w841:bool)
        n362 = case shown="True" w841 {
          frame False {
          }
          frame True {
            w846 = FALSE ("Ack hard alarm!")
            n363 = property on="Hard Alarm" class="Bool (strict)"("Value"=w846) -> ()  [unwired: 2 in, 2 out]
            n364 = property on="System Alarm" class="Bool (strict)"("Value"=w846) -> ()  [unwired: 2 in, 2 out]
            n365 = property on="System Alarm" class="Bool (strict)"("Value"=w846) -> ()  [unwired: 2 in, 2 out]
          }
        }
        n366 = case shown="True" "Acknowledge" {
          tunnel: [w844 0.0 ("Numeric")] -> w838
          tunnel: w839 -> [w844 _]
          frame False {
          }
          frame True {
          }
        }
      }
      frame True {
        n367 = local read "Table"() -> (w854:string[][])
        n368 = call "Error list.vi"("Error code"=w851, "Error array in"=w854) -> ("Hard alarm?"=w848:bool, "Error array out"=w853:string[][])  [unwired: 8 in]
        "Hard Alarm" <- w848
        n369 = Not(x=w848) -> (.not. x?=w849:bool)
        "Soft Alarm" <- w849
        n370 = Or(x=w849, y=w848) -> (x .or. y?=→"System Alarm":bool)
        n371 = case shown="True" w849 {
          frame False {
          }
          frame True {
            n372 = property on="Alarm ack" class="Bool"("DisabledEnum"=T11."Enabled" ("Disabled")) -> ()  [unwired: 2 in, 2 out]
          }
        }
        n373 = local write "Table"(w853) -> ()
        n374 = local write "Acknowledge"(FALSE ("Acknowledge")) -> ()
        n375 = property on="Tab Control" class="TabCtl (strict)"("Value"=6) -> ()  [unwired: 2 in, 2 out]
      }
    }
    n376 = case shown="1" w584 {
      tunnel: w533 -> [w814 w816 _ _]
      tunnel: w532 -> [_ w815 _ _]
      tunnel: [w814 w816 w817 w818] -> w470
      tunnel: [0.0 ("y") w815 w817 w818] -> w468
      frame 0, Default {
      }
      frame 1 {
      }
      frame 2 {
        w817 = 0.0 ("y")
      }
      frame 3 {
        w818 = 0.0 ("y")
      }
    }
    n377 = case shown="False" "Demo On" {
      tunnel: w494 -> [w700 _]
      tunnel: [w700 w732] -> w493
      tunnel: w492 -> [w699 _]
      tunnel: [w699 w702] -> w491
      tunnel: w490 -> [w698 _]
      tunnel: [w698 w709] -> _
      tunnel: w489 -> [w697 _]
      tunnel: [w697 w709] -> _
      tunnel: w488 -> [w696 _]
      tunnel: [w696 w709] -> _
      tunnel: w487 -> [w695 _]
      tunnel: [w695 w709] -> _
      tunnel: [w694 w730] -> w485
      tunnel: w486 -> [w694 _]
      tunnel: w484 -> [w693 _]
      tunnel: [w693 w709] -> _
      tunnel: w483 -> [w692 _]
      tunnel: [w692 w728] -> w482
      tunnel: w481 -> [w691 _]
      tunnel: [w691 w726] -> w480
      tunnel: w479 -> [w690 _]
      tunnel: [w690 w709] -> w478
      tunnel: w477 -> [w689 _]
      tunnel: [w689 w709] -> w476
      tunnel: w475 -> [w688 _]
      tunnel: [w688 w709] -> w474
      tunnel: w473 -> [w687 _]
      tunnel: [w687 w709] -> w472
      tunnel: w471 -> [_ w735]
      tunnel: w470 -> [w686 _]
      tunnel: [w686 w734] -> w469
      tunnel: w468 -> [w685 _]
      tunnel: [w685 w709] -> w467
      tunnel: w466 -> [w684 _]
      tunnel: [w684 w724] -> w465
      tunnel: w464 -> [w683 _]
      tunnel: [w683 w709] -> w463
      tunnel: w462 -> [w682 _]
      tunnel: [w682 w722] -> w461
      tunnel: w460 -> [w681 _]
      tunnel: [w681 w720] -> w459
      tunnel: w458 -> [w680 _]
      tunnel: [w680 w718] -> w457
      tunnel: w456 -> [w679 _]
      tunnel: [w679 w716] -> w455
      tunnel: w454 -> [w678 _]
      tunnel: [w678 w714] -> w453
      tunnel: w452 -> [w677 _]
      tunnel: [w677 w712] -> w451
      tunnel: w450 -> [w676 _]
      tunnel: [w676 w711] -> w449
      tunnel: w448 -> [w675 _]
      tunnel: [w675 w710] -> w447
      tunnel: w446 -> [w674 _]
      tunnel: [w674 w709] -> w445
      tunnel: w444 -> [w673 _]
      tunnel: [w673 w707] -> w443
      tunnel: w442 -> [w672 _]
      tunnel: [w672 w708] -> w441
      tunnel: w440 -> [w671 _]
      tunnel: [w671 w708] -> w439
      tunnel: w438 -> [w670 _]
      tunnel: [w670 w708] -> w437
      frame False {
      }
      frame True {
        w708 = 5.0 ("Numeric")
        w709 = 0.0 ("Numeric")
        n378 = Index Array(array=w735, index #1=2 ("index"), index #2=13 ("index"), index #3=14 ("index"), index #4=0 ("index"), index #5=1 ("index"), index #6=4 ("index"), index #7=5 ("index"), index #8=6 ("index"), index #9=7 ("index"), index #10=8 ("index"), index #11=9 ("index"), index #12=10 ("index"), index #13=11 ("index"), index #14=15 ("index"), index #15=3 ("index"), index #16=12 ("index")) -> (element #1=w734:dbl, element #2=w732:dbl, element #3=w730:dbl, element #4=w728:dbl, element #5=w726:dbl, element #6=w724:dbl, element #7=w722:dbl, element #8=w720:dbl, element #9=w718:dbl, element #10=w716:dbl, element #11=w714:dbl, element #12=w712:dbl, element #13=w711:dbl, element #14=w710:dbl, element #15=w707:dbl, element #16=w702:dbl)
      }
    }
    n379 = call "Flow_Guide-plot.vi"("Temperature Sync"="Flow Sync", "Temp Band % (e.g. 1%=1.01)"="Flow Band %", "Mean(Off)/Interval(On)"="Mean(Off)/Interval(On) 2", "Guide"="FlowGuide") -> ()  [unwired: 5 in, 3 out]
    n380 = Merge Signals(w485) -> (→"HC Concentration (ppm)":dynamicdata)
    n381 = Merge Signals(w465, w463, w461, w459, w457) -> (→"System Temperatures (°C)":dynamicdata)
    n382 = Merge Signals(w455, w453, w451, w449) -> (→"Heat Exchanger Temperatures (°C)":dynamicdata)
    n383 = Merge Signals(w447, w445) -> (→"NO Concentration (ppm)":dynamicdata)
    n384 = Merge Signals(w443, w441, w439, w437) -> (→"Lambda":dynamicdata)
    n385 = Merge Signals(w469, w467) -> (→"Flow Rate (g/s)":dynamicdata)
    n386 = Merge Signals(w493, w491) -> (→"O2/CO Concentration":dynamicdata)
    n387 = call "Temp_Guide-plot.vi"("Time In"=w530, "Temperature Sync"="Temperature Sync", "Temp Band % (e.g. 1%=1.01)"="Temp Band %", "Mean(Off)/Interval(On)"="Mean(Off)/Interval(On)", "TempGuide"="TempGuide") -> ("Graph 4"=w529:dbl, "Graph 3"=w528:dbl, "Graph 2"=w527:dbl, "Graph 1"=w526:dbl, "Time out"=w531:i32)  [unwired: 2 in]
    n388 = local read "stop 2"() -> (w632:bool)
    n389 = Merge Signals(w482, w480, w478, w476, w474, w472, w526, w527, w528, w529) -> (→"Sample Temperatures (°C)":dynamicdata)
    n390 = node-c288() -> ()  [unwired: 1 in, 1 out]
  }
  n391 = timed-loop {
    timing: w7 -> [_]
    timing-out: [_] -> w6
    stop <- _ stop-if-true
    n392 = node-c288() -> ()  [unwired: 1 in, 1 out]
    n393 = shared-variable "RT CompactRIO Target 2\\Library 1.lvlib\\DATA_2"() -> (w936:dbl[])  [unwired: 1 in, 1 out]
    n394 = Add(x=0 ("index"), y="MFC Number") -> (x+y=w953:i32)
    n395 = Add(x="MFC Number", y=8) -> (x+y=w952:i32)
    n396 = case shown="\"CO\", Default" "Graph 1 Box" {
      tunnel: [0 ("index") 1 ("index") 2 ("index") 3 ("index") 4 ("index") 5 ("index") 6 ("index") 7 ("index")] -> w937
      tunnel: [8 ("index") 9 ("index") 10 ("index") 11 ("index") 12 ("index") 13 ("index") 14 ("index") 15 ("index")] -> w944
      frame "CO", Default {
      }
      frame "HC Cycle 1" {
      }
      frame "Air Cycle 1" {
      }
      frame "NO" {
      }
      frame "Air Bal" {
      }
      frame "HC Bal" {
      }
      frame "Air Cycle 2" {
      }
      frame "HC Cycle 2" {
      }
    }
    n397 = case shown="\"Air Cycle 2\"" "Graph 2 Box" {
      tunnel: [0 ("index") 1 ("index") 2 ("index") 3 ("index") 4 ("index") 5 ("index") 6 ("index") 7 ("index")] -> w928
      tunnel: [8 ("index") 9 ("index") 10 ("index") 11 ("index") 12 ("index") 13 ("index") 14 ("index") 15 ("index")] -> w929
      frame "CO" {
      }
      frame "HC Cycle 1", Default {
      }
      frame "Air Cycle 1" {
      }
      frame "NO" {
      }
      frame "Air Bal" {
      }
      frame "HC Bal" {
      }
      frame "Air Cycle 2" {
      }
      frame "HC Cycle 2" {
      }
    }
    n398 = call "MKS.vi"("IP Address"="192.168.254.2" ("IP_ADD [127.0.0.1]"), "Connect"="MKS 5Hz") -> ("Emissions"=w945:dbl[])  [unwired: 9 in]
    n399 = Build Array (concatenate)(w936, w945) -> (w951:dbl[])
    n400 = for {
      tunnel: w951 -> [w1039] mode=indexing
      tunnel: [w1038] -> w961 mode=indexing
      n401 = Number To Fractional String(number=w1039, precision (6)=i16 3) -> (F-format string=w1038:string)  [unwired: 2 in]
    }
    n402 = case shown="\"Air Cycle 1\", Default" "Graph 3 Box" {
      tunnel: [0 ("index") 1 ("index") 2 ("index") 3 ("index") 4 ("index") 5 ("index") 6 ("index") 7 ("index")] -> w926
      tunnel: [8 ("index") 9 ("index") 10 ("index") 11 ("index") 12 ("index") 13 ("index") 14 ("index") 15 ("index")] -> w927
      frame "CO" {
      }
      frame "HC Cycle 1" {
      }
      frame "Air Cycle 1", Default {
      }
      frame "NO" {
      }
      frame "Air Bal" {
      }
      frame "HC Bal" {
      }
      frame "Air Cycle 2" {
      }
      frame "HC Cycle 2" {
      }
    }
    n403 = case shown="\"NO\", Default" "Graph 4 Box" {
      tunnel: [0 ("index") 1 ("index") 2 ("index") 3 ("index") 4 ("index") 5 ("index") 6 ("index") 7 ("index")] -> w924
      tunnel: [8 ("index") 9 ("index") 10 ("index") 11 ("index") 12 ("index") 13 ("index") 14 ("index") 15 ("index")] -> w925
      frame "CO" {
      }
      frame "HC Cycle 1" {
      }
      frame "Air Cycle 1" {
      }
      frame "NO", Default {
      }
      frame "Air Bal" {
      }
      frame "HC Bal" {
      }
      frame "Air Cycle 2" {
      }
      frame "HC Cycle 2" {
      }
    }
    n404 = Index Array(array=w936, index #1=w953, index #2=w952) -> (element #1=w958:dbl, element #2=w957:dbl)
    n405 = Get Date/Time In Seconds() -> (seconds since 1Jan1904=w964:timestamp)
    n406 = local read "File name"() -> (w968:string)
    n407 = Index Array(array=w945, index="HC Index") -> (element=→"MKS HC":dbl)
    n408 = Format Date/Time String(time format string (%c)="%d/%m/%y %H:%M:%S", seconds (now)=w964) -> (date/time string=w962:string)  [unwired: 1 in]
    n409 = Concatenate Strings(w968, "_MFC" ("string")) -> (w966:string)
    n410 = Index Array(array=w936, index #1=w937, index #2=w944) -> (element #1=w939:dbl, element #2=w938:dbl)
    n411 = Index Array(array=w936, index #1=w928, index #2=w929) -> (element #1=w935:dbl, element #2=w934:dbl)
    n412 = Index Array(array=w936, index #1=w926, index #2=w927) -> (element #1=w933:dbl, element #2=w932:dbl)
    n413 = Index Array(array=w936, index #1=w924, index #2=w925) -> (element #1=w931:dbl, element #2=w930:dbl)
    n414 = Build Array (concatenate)(w962, w961) -> (w960:string[])
    n415 = String To Path(string=w966) -> (path=w963:path)
    n416 = Merge Signals(w939, w938) -> (→"MFC Graph 1":dynamicdata)
    n417 = Merge Signals(w935, w934) -> (→"MFC Graph 2":dynamicdata)
    n418 = Merge Signals(w933, w932) -> (→"MFC Graph 3":dynamicdata)
    n419 = Merge Signals(w931, w930) -> (→"MFC Graph 4":dynamicdata)
    n420 = local read "Log?"() -> (w959:bool)
    n421 = case shown="True" w959 {
      tunnel: w963 -> [w1033 w1036]
      tunnel: [w1033 w1034] -> _
      tunnel: w960 -> [_ w1035]
      frame False {
      }
      frame True {
        n422 = call-poly <vilib>:"Write To Spreadsheet File.vi"("append to file? (new file:F)"=TRUE, "1D data"=w1035, "file path (dialog if empty)"=w1036) -> ("new file path (Not A Path if cancelled)"=w1034:path)  [unwired: 5 in]
      }
    }
    n423 = Merge Signals(w958, w957) -> (→"MFC Setpoint/Delivery":dynamicdata)
    n424 = node-c288() -> ()  [unwired: 1 in, 1 out]
  }
  n425 = while {
    tunnel: w41 -> [w1047]
    tunnel: w25 -> [w1045]
    tunnel: w27 -> [w1044]
    tunnel: [FALSE ("stop 2")] -> w15
    stop <- w1048 stop-if-true
    n426 = Dequeue Element(queue=w1047) -> (element=w1046:T10)  [unwired: 2 in, 3 out]
    n427 = case shown="\"Leak Test\"" w1046 {
      tunnel: w1045 -> [_ _ _ w1103 w1114 w1150 w1184 _ _ _ _ _ _ _ w1547 _ _ _ _ _ _ _ _]
      tunnel: w1044 -> [_ _ _ _ _ _ _ _ w1197 w1212 w1267 w1312 _ _ _ _ _ _ _ _ _ _ _]
      frame "main", Default {
        # "20"
        # "25"
        # "30"
        # "15"
        # "10"
        # "5"
        # "0"
        # "30"
        # "25"
        # "20"
        # "15"
        # "10"
        # "5"
        # "0"
        # "Output Cluster\n\n0 NOx Conc\n1 CO conc %\n2 HC conc %\n3 Bleed H2O \n4 Bleed CO2\n5 Bleed N2 \n6 lambda P\n7 lambda I\n8 lambda D\n9 purge duration\n10 Target furnace lambda\n11 HC reaction ct\n12 Full system\n13 Log interval\n14 MKS 1\n15 MKS 2"
        n428 = local read "output cluster"() -> (w1077:T2)
        n429 = Unbundle(w1077) -> ("NOx Concentration (ppm)"=w1063:T1, "CO concentration %"=w1062:T1, "HC concentration %"=w1061:T1, "Bleed H2O %"=w1060:T1, "Bleed CO2 %"=w1059:T1, "Bleed N2 %"=w1074:T1, "lambda P"=w1073:T1, "lambda I"=w1072:T1, "lambda D"=w1075:T1, "Purge duration (seconds)"=w1076:T1, "Target furnace lambda"=w1068:T1, "HC reaction constant"=w1067:T1, w1069:i16, "Log interval (HRS)"=→"Log interval (seconds)":T1, w1056:i16, w1055:i16, "Advanced Logging"=→"Advanced Logging":bool, "Cycle Length (Hours)"=w1053:T1, "Heat Load Control"=w1052:bool, w1050:T1[])
        n430 = local read "Test Flow Rate(g/s)"() -> (w1089:T1)
        n431 = local read "Test number"() -> (w1094:u16)
        n432 = local read "Inlet LAMBDA"() -> (w1081:T1)
        n433 = local read "NO ppm Loff"() -> (w1079:T1)
        n434 = local read "NO:CO Ratio"() -> (w1078:T1)
        n435 = local read "Inlet O2 (%)"() -> (w1080:T1)
        n436 = local read "Connected"() -> (w1083:bool)
        n437 = Boolean To (0,1)(Boolean=w1052) -> (0, 1=w1051:i16)
        n438 = Boolean To (0,1)(Boolean=w1083) -> (0, 1=w1066:i16)
        n439 = Build Array (concatenate)("Stop Cmd", w1094, w1089, "Test Start Temperature (°C)", "Test Stop temperature (°C)", "Furnace Ramp Rate (°C/min)", w1081, w1080, "Inlet LAMBDA Rich", "Inlet LAMBDA Lean", "Inlet Temperature (°C)", "NO ppm SW", w1079, w1078, "Temperature Limit (°C)", w1066, "Inlet temp Age", "Flow rate Age", w1063, w1062, w1061, w1060, w1059, w1074, w1073, w1072, w1075, w1076, w1068, w1067, w1069, w1053, w1051, w1050) -> (w1085:T1[])
        n440 = Not Equal To 0?(x=w1069) -> (x != 0?=→"Full system?":bool)
        n441 = shared-variable "RT CompactRIO Target 2\\Library 1.lvlib\\Control Variables"(w1085) -> ()  [unwired: 1 in, 1 out]
        n442 = Not Equal To 0?(x=w1056) -> (x != 0?=w1057:bool)
        "7170" <- w1057
        n443 = Not Equal To 0?(x=w1055) -> (x != 0?=w1049:bool)
        "MKS" <- w1049
        n444 = Or(x=w1057, y=w1049) -> (x .or. y?=→"Connected":bool)
      }
      frame "start test" {
        w1095 = FALSE
        n445 = property on="Pass" class="Bool (strict)"("Value"=w1095) -> ()  [unwired: 2 in, 2 out]
        n446 = property on="Fail" class="Bool (strict)"("Value"=w1095) -> ()  [unwired: 2 in, 2 out]
        n447 = local write "Pass"(w1095) -> ()
        n448 = local write "Fail"(w1095) -> ()
        n449 = shared-variable "RT CompactRIO Target 2\\Library 1.lvlib\\Enum 1"("Enum 1") -> ()  [unwired: 1 in, 1 out]
      }
      frame "clear table 1" {
        n450 = property on="Sub-Cycle Name" class="Str (strict)"("Value"="" ("Subcycle name")) -> ()  [unwired: 2 in, 2 out]
        n451 = local write "Flag1"(FALSE) -> ()
        n452 = local write "Sub-Cycle Pattern"(string[][] [["", "0", "", "", "", "", "", "", "", "", "", "", ""], ["", "", "", "", "", "", "", "", "", "", "", "", ""], ["", "", "", "", "", "", "", "", "", "", "", "", ""], ["", "", "", "", "", "", "", "", "", "", "", "", ""], ["", "", "", "", "", "", "", "", "", "", "", "", ""], ["", "", "", "", "", "", "", "", "", "", "", "", ""], ["", "", "", "", "", "", "", "", "", "", "", "", ""], ["", "", "", "", "", "", "", "", "", "", "", "", ""], ["", "", "", "", "", "", "", "", "", "", "", "", ""], ["", "", "", "", "", "", "", "", "", "", "", "", ""], ["", "", "", "", "", "", "", "", "", "", "", "", ""], ["", "", "", "", "", "", "", "", "", "", "", "", ""], ["", "", "", "", "", "", "", "", "", "", "", "", ""], ["", "", "", "", "", "", "", "", "", "", "", "", ""], ["", "", "", "", "", "", "", "", "", "", "", "", ""], ["", "", "", "", "", "", "", "", "", "", "", "", ""], ["", "", "", "", "", "", "", "", "", "", "", "", ""], ["", "", "", "", "", "", "", "", "", "", "", "", ""], ["", "", "", "", "", "", "", "", "", "", "", "", ""], ["", "", "", "", "", "", "", "", "", "", "", "", ""], ["", "", "", "", "", "", "", "", "", "", "", "", ""], ["", "", "", "", "", "", "", "", "", "", "", "", ""], ["", "", "", "", "", "", "", "", "", "", "", "", ""], ["", "", "", "", "", "", "", "", "", "", "", "", ""], ["", "", "", "", "", "", "", "", "", "", "", "", ""], ["", "", "", "", "", "", "", "", "", "", "", "", ""], ["", "", "", "", "", "", "", "", "", "", "", "", ""], ["", "", "", "", "", "", "", "", "", "", "", "", ""], ["", "", "", "", "", "", "", "", "", "", "", "", ""], ["", "", "", "", "", "", "", "", "", "", "", "", ""], ["", "", "", "", "", "", "", "", "", "", "", "", ""]]) -> ()
      }
      frame "update list 1" {
        n453 = String To Path(string=w1103) -> (path=w1102:path)
        n454 = List Folder(path=w1102, pattern="*.eyes") -> (filenames=w1101:string[])  [unwired: 2 in, 3 out]
        n455 = property on="Sub-Cycle List" class="LstBox (strict)"("Item Names"=w1101) -> ()  [unwired: 2 in, 2 out]
      }
      frame "save subc" {
        w1107 = ".eyes" ("string")
        n456 = local read "Sub-Cycle Name"() -> (w1106:T5)
        n457 = String To Path(string=w1114) -> (path=w1119:path)
        n458 = Equal?(x=w1106, y="") -> (x = y?=w1111:bool)
        n459 = List Folder(path=w1119, pattern="*.eyes" ("string")) -> (filenames=w1118:string[])  [unwired: 2 in, 3 out]
        n460 = Concatenate Strings(w1106, w1107) -> (w1105:string)
        n461 = Concatenate Strings(w1114, w1106, w1107) -> (w1120:string)
        n462 = Search 1D Array(1D array=w1118, element=w1105) -> (index of element=w1117:i32)  [unwired: 1 in]
        n463 = case shown="True" w1111 {
          tunnel: [TRUE FALSE] -> w1110
          frame False {
          }
          frame True {
            n464 = One Button Dialog(message="Insert file name!") -> ()  [unwired: 1 in, 1 out]
          }
        }
        n465 = String To Path(string=w1120) -> (path=w1113:path)
        n466 = Equal?(x=w1117, y=-1) -> (x = y?=w1115:bool)
        n467 = case shown="False" w1115 {
          selector: w1115 -> [_ w1126]
          tunnel: [w1124 w1126] -> w1109
          frame False {
            n468 = Two Button Dialog(message="A file with this name already exists!\nDo you want to overwrite?") -> (T button?=w1124:bool)  [unwired: 2 in]
          }
          frame True {
          }
        }
        n469 = And(x=w1109, y=w1110) -> (x .and. y?=w1108:bool)
        n470 = case shown="True" w1108 {
          tunnel: w1113 -> [_ w1131]
          frame False {
          }
          frame True {
            n471 = local read "Sub-Cycle Pattern"() -> (w1130:string[][])
            n472 = call "Table check.vi"("Input table"=w1130) -> ("Incomplete?"=w1128:bool, "Length"=w1129:i32)  [unwired: 9 in]
            n473 = case shown="False" w1128 {
              tunnel: w1130 -> [w1139 _]
              tunnel: w1131 -> [w1138 _]
              tunnel: w1129 -> [w1137 _]
              tunnel: string[] [] -> [w1136 _]
              frame False {
                n474 = for {
                  N: w1137 -> [_]
                  tunnel: w1139 -> [w1146]
                  shift-right: [w1143] -> w1135
                  shift-left: w1136 -> [w1144]
                  i -> [w1145]
                  n475 = Index Array(array=w1146, index (row)=w1145) -> (element=w1142:string[])  [unwired: 1 in]
                  n476 = Delete From Array(array=w1142, index=0) -> (array with subset deleted=w1141:string[])  [unwired: 1 in, 1 out]
                  n477 = Build Array (concatenate)(w1144, w1141) -> (w1143:string[])
                }
                n478 = Build Array (concatenate)("SubCycle Data File for EYECAT - do not modify", w1135) -> (w1133:string[])
                n479 = call-poly <vilib>:"Write To Spreadsheet File.vi"("1D data"=w1133, "file path (dialog if empty)"=w1138) -> ()  [unwired: 6 in, 1 out]
              }
              frame True {
                n480 = One Button Dialog(message="The table is incomplete!\nplease review and save again!") -> ()  [unwired: 1 in, 1 out]
              }
            }
            n481 = local write "Flag1"(FALSE) -> ()
          }
        }
      }
      frame "load subc" {
        n482 = local read "Flag1"() -> (w1151:bool)
        n483 = case shown="True" w1151 {
          tunnel: [w1178 w1180] -> w1149
          tunnel: w1150 -> [w1178 w1180]
          tunnel: [TRUE w1179] -> w1148
          frame False {
          }
          frame True {
            n484 = Two Button Dialog(message="The table has been modified.\nDo you want to continue?") -> (T button?=w1179:bool)  [unwired: 2 in]
          }
        }
        n485 = case shown="True" w1148 {
          tunnel: w1149 -> [_ w1155]
          frame False {
          }
          frame True {
            n486 = property on="Sub-Cycle List" class="LstBox (strict)"() -> ("Item Names"=w1167:string[])  [unwired: 2 in, 2 out]
            n487 = Index Array(array=w1167, index="Sub-Cycle List") -> (element=w1154:string)
            n488 = Concatenate Strings(w1155, w1154) -> (w1165:string)
            n489 = Search/Split String(string=w1154, search string/char (-)=".") -> (substring before match=w1152:string)  [unwired: 1 in, 2 out]
            n490 = local write "Sub-Cycle Name"(w1152) -> ()
            n491 = String To Path(string=w1165) -> (path=w1164:path)
            n492 = call-poly <vilib>:"Read From Spreadsheet File.vi"("file path (dialog if empty)"=w1164) -> ("first row"=w1160:string[])  [unwired: 6 in, 4 out]
            n493 = Delete From Array(array=w1160, length=1, index=0) -> (array with subset deleted=w1157:string[])  [unwired: 1 out]
            n494 = Array Size(array=w1157) -> (size(s)=w1163:i32)
            n495 = Divide(x=w1163, y=12) -> (x/y=w1156:dbl)
            n496 = for {
              N: w1156 -> [_]
              shift-right: [w1173] -> _
              shift-left: w1157 -> [w1176]
              tunnel: [w1172] -> w1161 mode=indexing
              i -> [w1171]
              n497 = Increment(x=w1171) -> (x+1=w1170:i32)
              n498 = Delete From Array(array=w1176, length=12, index=0) -> (deleted portion=w1168:string[], array with subset deleted=w1173:string[])
              n499 = Number To Decimal String(number=w1170) -> (decimal integer string=w1169:string)  [unwired: 1 in]
              n500 = Build Array (concatenate)(w1169, w1168) -> (w1172:string[])
            }
            n501 = local write "Sub-Cycle Pattern"(w1161) -> ()
          }
        }
      }
      frame "delete subc" {
        n502 = Two Button Dialog(message="This operation will permanently delete this file!\nDo you want to continue?") -> (T button?=w1183:bool)  [unwired: 2 in]
        n503 = case shown="True" w1183 {
          tunnel: w1184 -> [_ w1189]
          frame False {
          }
          frame True {
            n504 = local read "Sub-Cycle List"() -> (w1186:i32)
            n505 = property on="Sub-Cycle List" class="LstBox (strict)"() -> ("Item Names"=w1187:string[])  [unwired: 2 in, 2 out]
            n506 = Index Array(array=w1187, index=w1186) -> (element=w1191:string)
            n507 = Concatenate Strings(w1189, w1191) -> (w1190:string)
            n508 = local write "Flag1"(FALSE) -> ()
            n509 = String To Path(string=w1190) -> (path=w1188:path)
            n510 = Delete(path (use dialog)=w1188) -> ()  [unwired: 4 in, 3 out]
          }
        }
      }
      frame "clear table 2" {
        n511 = property on="Cycle Name" class="Str (strict)"("Value"="" ("Subcycle name")) -> ()  [unwired: 2 in, 2 out]
        n512 = local write "Flag 2"(FALSE) -> ()
        n513 = local write "Cycle Pattern"(string[][] [["", "", "", "", ""], ["", "", "", "", ""], ["", "", "", "", ""], ["", "", "", "", ""], ["", "", "", "", ""], ["", "", "", "", ""], ["", "", "", "", ""], ["", "", "", "", ""], ["", "", "", "", ""], ["", "", "", "", ""], ["", "", "", "", ""], ["", "", "", "", ""], ["", "", "", "", ""], ["", "", "", "", ""], ["", "", "", "", ""], ["", "", "", "", ""], ["", "", "", "", ""], ["", "", "", "", ""], ["", "", "", "", ""], ["", "", "", "", ""], ["", "", "", "", ""], ["", "", "", "", ""], ["", "", "", "", ""], ["", "", "", "", ""], ["", "", "", "", ""], ["", "", "", "", ""], ["", "", "", "", ""], ["", "", "", "", ""], ["", "", "", "", ""], ["", "", "", "", ""], ["", "", "", "", ""]]) -> ()
      }
      frame "update list 2" {
        n514 = String To Path(string=w1197) -> (path=w1198:path)
        n515 = List Folder(path=w1198, pattern="*.eyec") -> (filenames=w1196:string[])  [unwired: 2 in, 3 out]
        n516 = property on="Cycle List" class="LstBox (strict)"("Item Names"=w1196) -> ()  [unwired: 2 in, 2 out]
      }
      frame "save cycle" {
        w1199 = ".eyec" ("string")
        n517 = local read "Cycle Name"() -> (w1200:T5)
        n518 = String To Path(string=w1212) -> (path=w1213:path)
        n519 = List Folder(path=w1213, pattern="*.eyec" ("string")) -> (filenames=w1211:string[])  [unwired: 2 in, 3 out]
        n520 = Equal?(x=w1200, y="") -> (x = y?=w1206:bool)
        n521 = Concatenate Strings(w1200, w1199) -> (w1202:string)
        n522 = Search 1D Array(1D array=w1211, element=w1202) -> (index of element=w1210:i32)  [unwired: 1 in]
        n523 = Concatenate Strings(w1212, w1200, w1199) -> (w1215:string)
        n524 = case shown="True" w1206 {
          tunnel: [TRUE FALSE] -> w1204
          frame False {
          }
          frame True {
            n525 = One Button Dialog(message="Insert file name!") -> ()  [unwired: 1 in, 1 out]
          }
        }
        n526 = String To Path(string=w1215) -> (path=w1214:path)
        n527 = Equal?(x=w1210, y=-1) -> (x = y?=w1208:bool)
        n528 = case shown="False" w1208 {
          selector: w1208 -> [_ w1264]
          tunnel: [w1262 w1264] -> w1205
          frame False {
            n529 = Two Button Dialog(message="A file with this name already exists!\nDo you want to overwrite?") -> (T button?=w1262:bool)  [unwired: 2 in]
          }
          frame True {
          }
        }
        n530 = And(x=w1205, y=w1204) -> (x .and. y?=w1203:bool)
        n531 = case shown="True" w1203 {
          tunnel: w1214 -> [_ w1222]
          frame False {
          }
          frame True {
            n532 = local read "Cycle Pattern"() -> (w1221:string[][])
            n533 = call "Table check.vi"("Input table"=w1221) -> ("Incomplete?"=w1219:bool, "Length"=w1220:i32)  [unwired: 9 in]
            n534 = case shown="False" w1219 {
              tunnel: w1222 -> [w1231 _]
              tunnel: w1221 -> [w1230 _]
              tunnel: w1220 -> [w1223 _]
              frame False {
                n535 = Number To Decimal String(number=w1223) -> (decimal integer string=w1226:string)  [unwired: 1 in]
                n536 = for {
                  N: w1223 -> [_]
                  tunnel: w1230 -> [w1260]
                  shift-right: [w1248] -> w1227
                  shift-left: string[] [] -> [w1258]
                  i -> [w1259]
                  w1239 = 12 ("length")
                  n537 = Index Array(array=w1260, index (row)=w1259) -> (element=w1254:string[])  [unwired: 1 in]
                  n538 = Index Array(array=w1254, index=3) -> (element=w1244:string)
                  n539 = Index Array(array=w1254, index=1) -> (element=w1243:string)
                  n540 = Concatenate Strings("C:\\Setup Files\\Subcycles Folder\\", w1243) -> (w1255:string)
                  n541 = String To Path(string=w1255) -> (path=w1256:path)
                  n542 = call-poly <vilib>:"Read From Spreadsheet File.vi"("file path (dialog if empty)"=w1256) -> ("first row"=w1247:string[])  [unwired: 6 in, 4 out]
                  n543 = Delete From Array(array=w1247, length=1, index=0) -> (array with subset deleted=w1241:string[])  [unwired: 1 out]
                  n544 = String Length(string=w1241) -> (length=w1250:i32[])
                  n545 = Array Size(array=w1250) -> (size(s)=w1242:i32)
                  n546 = Divide(x=w1242, y=w1239) -> (x/y=w1240:dbl)
                  n547 = Decrement(x=w1240) -> (x-1=w1232:dbl)
                  n548 = Multiply(x=w1239, y=w1232) -> (x*y=w1238:dbl)
                  n549 = Number To Decimal String(number=w1232) -> (decimal integer string=w1249:string)  [unwired: 1 in]
                  n550 = Delete From Array(array=w1241, length=12, index=w1238) -> (deleted portion=w1235:string[], array with subset deleted=w1236:string[])
                  n551 = Index Array(array=w1235, index=0) -> (element=w1233:string)
                  n552 = Build Array (concatenate)(w1243, w1244, w1249, w1233, w1236) -> (w1253:string[])
                  n553 = Build Array (concatenate)(w1258, w1253) -> (w1248:string[])
                }
                n554 = local write "Flag 2"(FALSE) -> ()
                n555 = Build Array (concatenate)("Cycle Data File for EYECAT - do not modify", w1226, w1227) -> (w1228:string[])
                n556 = call-poly <vilib>:"Write To Spreadsheet File.vi"("1D data"=w1228, "file path (dialog if empty)"=w1231) -> ()  [unwired: 6 in, 1 out]
              }
              frame True {
                n557 = One Button Dialog(message="The table is incomplete!\nplease review and save again!") -> ()  [unwired: 1 in, 1 out]
              }
            }
          }
        }
      }
      frame "load cycle" {
        n558 = local read "Flag 2"() -> (w1268:bool)
        n559 = case shown="True" w1268 {
          tunnel: [w1307 w1309] -> w1265
          tunnel: w1267 -> [w1307 w1309]
          tunnel: [TRUE ("T button?") w1308] -> w1266
          frame False {
          }
          frame True {
            n560 = Two Button Dialog(message="The table has been modified.\nDo you want to continue?") -> (T button?=w1308:bool)  [unwired: 2 in]
          }
        }
        n561 = case shown="True" w1266 {
          tunnel: w1265 -> [_ w1271]
          frame False {
          }
          frame True {
            n562 = property on="Cycle List" class="LstBox (strict)"() -> ("Item Names"=w1287:string[])  [unwired: 2 in, 2 out]
            n563 = Index Array(array=w1287, index="Cycle List") -> (element=w1273:string)
            n564 = Concatenate Strings(w1271, w1273) -> (w1286:string)
            n565 = Search/Split String(string=w1273, search string/char (-)=".") -> (substring before match=w1272:string)  [unwired: 1 in, 2 out]
            n566 = String To Path(string=w1286) -> (path=w1285:path)
            n567 = local write "Cycle Name"(w1272) -> ()
            n568 = call-poly <vilib>:"Read From Spreadsheet File.vi"("file path (dialog if empty)"=w1285) -> ("first row"=w1269:string[])  [unwired: 6 in, 4 out]
            n569 = Delete From Array(array=w1269, length=2, index=0) -> (array with subset deleted=w1270:string[])  [unwired: 1 out]
            n570 = Index Array(array=w1269, index=1) -> (element=w1284:string)
            n571 = Decimal String To Number(string=w1284) -> (number=w1283:i32)  [unwired: 2 in, 1 out]
            n572 = for {
              N: w1283 -> [_]
              tunnel: w1270 -> [w1305]
              tunnel: [w1300] -> w1278 mode=indexing
              shift-right: [w1290] -> _
              shift-left: 0 ("x") -> [w1291]
              i -> [w1304]
              w1301 = ""
              n573 = Increment(x=w1291) -> (x+1=w1289:i32)
              n574 = Increment(x=w1289) -> (x+1=w1297:i32)
              n575 = Increment(x=w1304) -> (x+1=w1299:i32)
              n576 = Number To Decimal String(number=w1299) -> (decimal integer string=w1298:string)  [unwired: 1 in]
              n577 = Index Array(array=w1305, index #1=w1291, index #2=w1289, index #3=w1297) -> (element #1=w1303:string, element #2=w1302:string, element #3=w1296:string)
              n578 = Build Array(w1298, w1303, w1301, w1302, w1301) -> (w1300:string[])
              n579 = Decimal String To Number(string=w1296) -> (number=w1295:i32)  [unwired: 2 in, 1 out]
              n580 = Multiply(x=w1295, y=12 ("x")) -> (x*y=w1293:i32)
              n581 = Compound Arithmetic op=ADD(w1293, 4, w1291) -> (w1290:i32)
            }
            n582 = Insert Into Array(array=string[][] [["", "", "", "", ""], ["", "", "", "", ""], ["", "", "", "", ""], ["", "", "", "", ""], ["", "", "", "", ""], ["", "", "", "", ""], ["", "", "", "", ""], ["", "", "", "", ""], ["", "", "", "", ""], ["", "", "", "", ""], ["", "", "", "", ""], ["", "", "", "", ""], ["", "", "", "", ""], ["", "", "", "", ""], ["", "", "", "", ""], ["", "", "", "", ""], ["", "", "", "", ""], ["", "", "", "", ""], ["", "", "", "", ""], ["", "", "", "", ""], ["", "", "", "", ""], ["", "", "", "", ""], ["", "", "", "", ""], ["", "", "", "", ""], ["", "", "", "", ""], ["", "", "", "", ""], ["", "", "", "", ""], ["", "", "", "", ""], ["", "", "", "", ""], ["", "", "", "", ""], ["", "", "", "", ""]], index (row)=0, new element=w1278) -> (w1277:string[][])  [unwired: 1 in]
            n583 = local write "Cycle Pattern"(w1277) -> ()
          }
        }
      }
      frame "delete cycle" {
        n584 = Two Button Dialog(message="This operation will permanently delete this file!\nDo you want to continue?") -> (T button?=w1313:bool)  [unwired: 2 in]
        n585 = case shown="True" w1313 {
          tunnel: w1312 -> [_ w1318]
          frame False {
          }
          frame True {
            n586 = local read "Cycle List"() -> (w1319:i32)
            n587 = property on="Cycle List" class="LstBox (strict)"() -> ("Item Names"=w1320:string[])  [unwired: 2 in, 2 out]
            n588 = Index Array(array=w1320, index=w1319) -> (element=w1317:string)
            n589 = Concatenate Strings(w1318, w1317) -> (w1316:string)
            n590 = String To Path(string=w1316) -> (path=w1315:path)
            n591 = Delete(path (use dialog)=w1315) -> ()  [unwired: 4 in, 3 out]
            n592 = local write "Flag 2"(FALSE) -> ()
          }
        }
      }
      frame "calc HC CO" {
        n593 = local read "Sub-Cycle Pattern"() -> (w1337:string[][])
        n594 = Index Array(array=w1337, index (col) #1=3 ("disabled index (col)"), index (col) #2=4 ("index (col)"), index (col) #3=11 ("index (col)")) -> (element #1=w1327:string[], element #2=w1334:string[], element #3=w1321:string[])  [unwired: 3 in]
        n595 = Array Size(array=w1327) -> (size(s)=w1325:i32)
        n596 = Search 1D Array(1D array=w1327, element="") -> (index of element=w1324:i32)  [unwired: 1 in]
        n597 = Equal?(x=w1324, y=-1) -> (x = y?=w1326:bool)
        n598 = Select(t=w1325, s=w1326, f=w1324) -> (s? t:f=w1323:i32)
        n599 = for {
          N: w1323 -> [_]
          tunnel: [w1348] -> w1331 mode=indexing
          tunnel: [w1347] -> w1330 mode=indexing
          tunnel: w1327 -> [w1346] mode=indexing
          tunnel: w1334 -> [w1345] mode=indexing
          tunnel: w1321 -> [w1344] mode=indexing
          w1343 = ""
          n600 = Not Equal?(x=w1346, y=w1343) -> (x != y?=w1342:bool)
          n601 = Not Equal?(x=w1345, y=w1343) -> (x != y?=w1341:bool)
          n602 = Not Equal?(x=w1344, y=w1343) -> (x != y?=w1340:bool)
          n603 = Compound Arithmetic op=AND(w1342, w1341, w1340) -> (w1339:bool)
          n604 = case shown="True" w1339 {
            tunnel: w1346 -> [_ w1377]
            tunnel: w1345 -> [_ w1376]
            tunnel: [w1349 w1373] -> w1347
            tunnel: [w1349 w1372] -> w1348
            tunnel: w1344 -> [_ w1350]
            frame False {
              w1349 = ""
            }
            frame True {
              # "O2Eq"
              n605 = Fract/Exp String To Number(string=w1350) -> (number=w1351:dbl)  [unwired: 3 in, 1 out]
              n606 = Fract/Exp String To Number(string=w1377) -> (number=w1358:dbl)  [unwired: 3 in, 1 out]
              n607 = Fract/Exp String To Number(string=w1376) -> (number=w1354:dbl)  [unwired: 3 in, 1 out]
              n608 = Decrement(x=w1358) -> (x-1=w1359:dbl)
              n609 = Divide(x=w1351, y=20000.0) -> (x/y=w1352:dbl)
              n610 = Multiply(x=4.76, y=w1358) -> (x*y=w1363:dbl)
              n611 = Multiply(x=w1359, y=100.0) -> (x*y=w1361:dbl)
              n612 = Add(x=w1354, y=w1352) -> (x+y=w1355:dbl)
              n613 = Add(x=0.33, y=w1363) -> (x+y=w1365:dbl)
              n614 = Divide(x=w1361, y=w1365) -> (x/y=w1366:dbl)
              n615 = Subtract(x=w1355, y=w1366) -> (x-y=w1368:dbl)
              n616 = Multiply(x=w1368, y=2.0) -> (x*y=w1356:dbl)
              n617 = Divide(x=w1368, y=5.0) -> (x/y=w1357:dbl)
              n618 = Number To Fractional String(number=w1357, width (-)=i16 6, precision (6)=i16 3) -> (F-format string=w1372:string)  [unwired: 1 in]
              n619 = Number To Fractional String(number=w1356, width (-)=i16 6, precision (6)=i16 2) -> (F-format string=w1373:string)  [unwired: 1 in]
            }
          }
        }
        n620 = Replace Array Subset(array=w1337, new element #1=w1331, index (col) #1=5 ("disabled index (col)"), new element #2=w1330, index (col) #2=6 ("disabled index (col)")) -> (w1335:string[][])  [unwired: 2 in]
        n621 = local write "Sub-Cycle Pattern"(w1335) -> ()
      }
      frame "Total time calc" {
        w1392 = i16 2 ("width (-)")
        w1399 = ":"
        n622 = local read "Cycle Pattern"() -> (w1406:string[][])
        n623 = Index Array(array=w1406, index (col)=4 ("disabled index (col)")) -> (element=w1379:string[])  [unwired: 1 in]
        n624 = Array Size(array=w1379) -> (size(s)=w1381:i32)
        n625 = Search 1D Array(1D array=w1379, element="") -> (index of element=w1380:i32)  [unwired: 1 in]
        n626 = Equal?(x=w1380, y=-1) -> (x = y?=w1382:bool)
        n627 = Select(t=w1381, s=w1382, f=w1380) -> (s? t:f=w1378:i32)
        n628 = for {
          N: w1378 -> [_]
          tunnel: w1379 -> [w1414] mode=indexing
          shift-right: [w1416] -> w1402
          shift-left: 0 -> [w1417]
          n629 = xnode "Match Regular Expression"("input string"=w1414, "regular expression"=":" ("search string/char (-)")) -> ("before match"=w1413:string, "after match"=w1410:string)  [unwired: 4 in, 3 out]
          n630 = Decimal String To Number(string=w1413) -> (number=w1412:i32)  [unwired: 2 in, 1 out]
          n631 = Decimal String To Number(string=w1410) -> (number=w1409:i32)  [unwired: 2 in, 1 out]
          n632 = Multiply(x=w1412, y=60) -> (x*y=w1408:i32)
          n633 = Add(x=w1408, y=w1409) -> (x+y=w1407:i32)
          n634 = Add(x=w1407, y=w1417) -> (x+y=w1416:i32)
        }
        n635 = local read "Total Number of Cycles"() -> (w1403:T1)
        n636 = Multiply(x=w1402, y=w1403) -> (x*y=w1398:T1)
        n637 = Quotient & Remainder(x=w1398, y=3600.0) -> (x-y*floor(x/y)=w1385:T1, floor(x/y)=w1395:T1)
        n638 = Quotient & Remainder(x=w1385, y=60.0) -> (x-y*floor(x/y)=w1393:T1, floor(x/y)=w1394:T1)
        n639 = Number To Decimal String(number=w1395) -> (decimal integer string=w1400:string)  [unwired: 1 in]
        n640 = Number To Decimal String(number=w1394, width (-)=w1392) -> (decimal integer string=w1396:string)
        n641 = Number To Decimal String(number=w1393, width (-)=w1392) -> (decimal integer string=w1391:string)
        n642 = Concatenate Strings(w1400, w1399, w1396, w1399, w1391) -> (w1390:string)
        n643 = call <vilib>:"Search and Replace Pattern.vi"("string"=w1390, "regular expression (\"\")"=" " ("replace string (\"\")"), "replace string (\"\")"="0" ("replace string (\"\")"), "replace all? (F)"=TRUE) -> ("result string"=→"Total Test Duration (hrs)":string)  [unwired: 1 in, 1 out]
      }
      frame "update Cycle pattern " {
        n644 = local read "Cycle Pattern"() -> (w1545:string[][])
        n645 = Index Array(array=w1545, index (col)=1 ("disabled index (col)")) -> (element=w1530:string[])  [unwired: 1 in]
        n646 = String To Path(string=w1547) -> (path=w1548:path)
        n647 = Array Size(array=w1530) -> (size(s)=w1533:i32)
        n648 = Search 1D Array(1D array=w1530, element="") -> (index of element=w1532:i32)  [unwired: 1 in]
        n649 = List Folder(path=w1548, pattern="*.eyes") -> (filenames=w1546:string[])  [unwired: 2 in, 3 out]
        n650 = Equal?(x=w1532, y=-1) -> (x = y?=w1534:bool)
        n651 = Select(t=w1533, s=w1534, f=w1532) -> (s? t:f=w1531:i32)
        n652 = for {
          N: w1531 -> [_]
          tunnel: w1545 -> [w1564] mode=indexing
          tunnel: w1547 -> [w1557]
          tunnel: [w1559] -> w1540 mode=indexing
          tunnel: [w1561] -> w1544 mode=indexing
          tunnel: [w1558] -> w1541 mode=indexing
          tunnel: w1546 -> [w1556]
          tunnel: [w1551] -> w1537 mode=indexing
          n653 = Index Array(array=w1564, index #1=1 ("index"), index #2=3 ("index")) -> (element #1=w1555:string, element #2=w1560:string)
          n654 = Search 1D Array(1D array=w1556, element=w1555) -> (index of element=w1554:i32)  [unwired: 1 in]
          n655 = Not Equal?(x=w1554, y=-1) -> (x != y?=w1552:bool)
          n656 = case shown="True" w1552 {
            tunnel: [w1568 w1582] -> w1561
            tunnel: w1560 -> [_ w1578]
            tunnel: [w1568 w1576] -> w1559
            tunnel: [w1568 w1575] -> w1558
            tunnel: w1557 -> [_ w1574]
            tunnel: w1555 -> [w1567 w1573]
            tunnel: [w1566 w1573] -> w1551
            frame False {
              w1568 = "N/A" ("String")
              n657 = Concatenate Strings(w1567, " - File NOT AVAILABLE !!!" ("string")) -> (w1566:string)
            }
            frame True {
              w1586 = i16 2 ("width (-)")
              n658 = Concatenate Strings(w1574, w1573) -> (w1604:string)
              n659 = String To Path(string=w1604) -> (path=w1603:path)
              n660 = call <vilib>:"Search and Replace Pattern.vi"("string"=w1578, "regular expression (\"\")"="[a-x ]" ("format string"), "replace string (\"\")"="", "replace all? (F)"=TRUE) -> ("result string"=w1575:string)  [unwired: 1 in, 1 out]
              n661 = call-poly <vilib>:"Read From Spreadsheet File.vi"("file path (dialog if empty)"=w1603) -> ("first row"=w1572:string[])  [unwired: 6 in, 4 out]
              n662 = Delete From Array(array=w1572, length=1, index=0) -> (array with subset deleted=w1571:string[])  [unwired: 1 out]
              n663 = Array Size(array=w1571) -> (size(s)=w1602:i32)
              n664 = Equal?(x=w1575, y="") -> (x = y?=w1590:bool)
              n665 = Subtract(x=w1602, y=12) -> (x-y=w1600:i32)
              n666 = Select(t="0", s=w1590, f=w1575) -> (s? t:f=w1589:string)
              n667 = Index Array(array=w1571, index=w1600) -> (element=w1576:string)
              n668 = Decimal String To Number(string=w1589) -> (number=w1599:i32)  [unwired: 2 in, 1 out]
              n669 = Decimal String To Number(string=w1576) -> (number=w1598:i32)  [unwired: 2 in, 1 out]
              n670 = Multiply(x=w1599, y=w1598) -> (x*y=w1597:i32)
              n671 = Quotient & Remainder(x=w1597, y=60) -> (x-y*floor(x/y)=w1595:i32, floor(x/y)=w1594:i32)
              n672 = Number To Decimal String(number=w1595, width (-)=w1586) -> (decimal integer string=w1592:string)
              n673 = Number To Decimal String(number=w1594, width (-)=w1586) -> (decimal integer string=w1591:string)
              n674 = Concatenate Strings(w1591, ":", w1592) -> (w1585:string)
              n675 = call <vilib>:"Search and Replace Pattern.vi"("string"=w1585, "regular expression (\"\")"=" " ("replace string (\"\")"), "replace string (\"\")"="0" ("replace string (\"\")"), "replace all? (F)"=TRUE) -> ("result string"=w1582:string)  [unwired: 1 in, 1 out]
            }
          }
        }
        n676 = Replace Array Subset(array=w1545, new element #1=w1537, index (col) #1=1 ("disabled index (col)"), new element #2=w1540, index (col) #2=2 ("disabled index (col)"), new element #3=w1541, index (col) #3=3 ("disabled index (col)"), new element #4=w1544, index (col) #4=4 ("disabled index (col)")) -> (w1549:string[][])  [unwired: 4 in]
        n677 = local write "Cycle Pattern"(w1549) -> ()
      }
      frame "load cycle name" {
        n678 = property on="Cycle Pattern" class="Tbl (strict)"() -> ("EditPos"=w1610:T3)  [unwired: 2 in, 2 out]
        n679 = Unbundle By Name(w1610) -> ("Row"=w1608:i32, "Column"=w1607:i32)
        n680 = local read "Cycle Pattern"() -> (w1606:string[][])
        n681 = call "SubCycles list.vi"() -> ("Subcycle name"=w1609:string)  [unwired: 10 in, 1 out]
        n682 = Replace Array Subset(array=w1606, new element=w1609, index (row)=w1608, index (col)=w1607) -> (w1605:string[][])
        n683 = local write "Cycle Pattern"(w1605) -> ()
      }
      frame "load test array" {
        n684 = local read "Total Test Duration (hrs)"() -> (w1618:T8)
        n685 = local read "Cycle Name"() -> (w1614:T5)
        n686 = Equal?(x=w1614, y="") -> (x = y?=w1613:bool)
        n687 = Not Equal?(x=w1618, y="0:00:00") -> (x != y?=w1612:bool)
        n688 = Or(x=w1612, y=w1613) -> (x .or. y?=w1611:bool)
        n689 = case shown="True" w1611 {
          selector: w1611 -> [w1619 _]
          tunnel: [FALSE TRUE] -> w1616
          frame False {
            n690 = case shown="False" w1619 {
              frame False {
                n691 = One Button Dialog(message="Incomplete Data!\nReview the cycle pattern!") -> ()  [unwired: 1 in, 1 out]
              }
              frame True {
              }
            }
          }
          frame True {
            w1625 = 0.0 ("default (0 I32)")
            n692 = local read "Cycle Name"() -> (w1640:T5)
            n693 = Concatenate Strings("C:\\Setup Files\\Cycles Folder\\", w1640, ".eyec" ("string")) -> (w1638:string)
            n694 = String To Path(string=w1638) -> (path=w1639:path)
            n695 = local read "Total Number of Cycles"() -> (w1636:T1)
            n696 = call-poly <vilib>:"Read From Spreadsheet File.vi"("file path (dialog if empty)"=w1639) -> ("first row"=w1622:string[])  [unwired: 6 in, 4 out]
            n697 = call "Remove names.vi"("Array in"=w1622) -> ("Array out"=w1631:string[])  [unwired: 10 in]
            n698 = Index Array(array=w1622, index #1=14 ("index"), index #2=15 ("index")) -> (element #1=w1627:string, element #2=w1623:string)
            n699 = Number To Decimal String(number="Ageing Gas") -> (decimal integer string=w1635:string)  [unwired: 1 in]
            n700 = Number To Decimal String(number=w1636) -> (decimal integer string=w1634:string)  [unwired: 1 in]
            n701 = Decimal String To Number(string=w1623, default (0L)=w1625) -> (number=w1624:dbl)  [unwired: 1 in, 1 out]
            n702 = Decimal String To Number(string=w1627, default (0L)=w1625) -> (number=w1626:dbl)  [unwired: 1 in, 1 out]
            n703 = property on="Inlet temp Age" class="DigNum (strict)"("Value"=w1626) -> ()  [unwired: 2 in, 2 out]
            n704 = property on="Flow rate Age" class="DigNum (strict)"("Value"=w1624) -> ()  [unwired: 2 in, 2 out]
            n705 = Build Array (concatenate)(w1635, w1634, w1631) -> (w1630:string[])
            n706 = shared-variable "RT CompactRIO Target 2\\Library 1.lvlib\\Ageing Variables"(w1630) -> ()  [unwired: 1 in, 1 out]
          }
        }
        "Test Compiled" <- w1616
      }
      frame "convert to num" {
        n707 = local read "EditPos Subc"() -> (w1645:T3)
        n708 = Unbundle By Name(w1645) -> ("Row"=w1646:i32, "Column"=w1643:i32)
        n709 = Equal?(x=w1643, y=7) -> (x = y?=w1642:bool)
        n710 = case shown="False" w1642 {
          tunnel: w1646 -> [_ w1651]
          tunnel: w1643 -> [_ w1649]
          tunnel: w1645 -> [_ _]
          frame True {
          }
          frame False {
            n711 = local read "Sub-Cycle Pattern"() -> (w1648:string[][])
            n712 = call "Conv to num.vi"("Column"=w1649, "Row"=w1651, "Array"=w1648) -> ("result string"=w1650:string)  [unwired: 8 in]
            n713 = Replace Array Subset(array=w1648, new element=w1650, index (row)=w1651, index (col)=w1649) -> (w1647:string[][])
            n714 = local write "Sub-Cycle Pattern"(w1647) -> ()
          }
        }
      }
      frame "check scycle name" {
        n715 = local read "Sub-Cycle Name"() -> (w1652:T5)
        n716 = call <vilib>:"Search and Replace Pattern.vi"("string"=w1652, "regular expression (\"\")"="[^0-9a-zA-Z ]" ("format string"), "replace string (\"\")"="", "replace all? (F)"=TRUE) -> ("result string"=w1658:string)  [unwired: 1 in, 1 out]
        n717 = Not Equal?(x=w1658, y=w1652) -> (x != y?=w1657:bool)
        n718 = case shown="False" w1657 {
          tunnel: w1658 -> [w1659 w1660]
          tunnel: [w1659 w1660] -> w1653
          frame False {
          }
          frame True {
            n719 = One Button Dialog(message="Unsuitable character for the file name!") -> ()  [unwired: 1 in, 1 out]
          }
        }
        n720 = local write "Sub-Cycle Name"(w1653) -> ()
      }
      frame "check cycle name" {
        n721 = local read "Cycle Name"() -> (w1662:T5)
        n722 = call <vilib>:"Search and Replace Pattern.vi"("string"=w1662, "regular expression (\"\")"="[^0-9a-zA-Z ]" ("format string"), "replace string (\"\")"="", "replace all? (F)"=TRUE) -> ("result string"=w1668:string)  [unwired: 1 in, 1 out]
        n723 = Not Equal?(x=w1668, y=w1662) -> (x != y?=w1667:bool)
        n724 = case shown="False" w1667 {
          tunnel: w1668 -> [w1669 w1670]
          tunnel: [w1669 w1670] -> w1663
          frame False {
          }
          frame True {
            n725 = One Button Dialog(message="Unsuitable character for the file name!") -> ()  [unwired: 1 in, 1 out]
          }
        }
        n726 = local write "Cycle Name"(w1663) -> ()
      }
      frame "Multigas connect" {
        # "add here logic to verify the user requirements and the machine state\n0 - not connected\n1 - MKS1 & Ext An Up\n2 - MKS2 & Ext An Dn\n3 - MKS 1 & 2  & Ext An Up & Dn"
        n727 = flat-sequence {
          frame #0 {
            "Connected?" <- TRUE
          }
        }
      }
      frame "Multigas disconnect" {
      }
      frame "Leak Test" {
        n728 = call "Press_Test.vi"() -> ("Reset Button"=w1673:bool)  [unwired: 11 in]
        n729 = local write "Leak Test"(w1673) -> ()
      }
    }
    n730 = local read "stop 2"() -> (w1048:bool)
  }
  n731 = node-c288(w6) -> ()  [unwired: 1 out]
  n732 = local write "stop 2"(w15) -> ()
  n733 = node-c288(w13) -> ()  [unwired: 1 out]
  "Table" <- string[][] [] ("Table")
